vi "Main_Marvin.vi"() -> ()   [LabVIEW 2017]
uses:
  PCAN_Driver/ControlCAN.llb/DevType.ctl
  PCAN_Driver/ControlCAN.llb/CAN Channel.ctl
  PCAN_Driver/ControlCAN.llb/VCI_INIT_CONFIG.ctl
  PCAN_Driver/ControlCAN.llb/InitFlag.ctl
  PCAN_Driver/ControlCAN.llb/Fliter.ctl
  PCAN_Driver/ControlCAN.llb/Mode.ctl
  <vilib>/Utility/miscctls.llb/LVRowAndColumnTypeDef.ctl
  <vilib>/Utility/cursorutil.llb/Set Cursor (Icon Pict).vi
  PCAN_Driver/ControlCAN.lvlib
panel:
  in  "Stop Burn-in":bool
  out "Array 2":dbl[](array[numeric])
  out "VISA resource name out":refnum<visa-resource-name>
  out "UUT":u8
  out "CAN Status":bool
  in  "Channel 2":T1 caption="Channel" items=["Channel 1", "Channel 2"]
  out "Config_CANAT":T7 {"DevType" items=["USB-CAN"=3, "USB-CAN2"=4]; "CanIndex" items=["通道1", "通道2"]; "VCI_INIT_CONFIG"."Fliter" items=["接收所有类型"=3, "只接收标准帧"=4, "只接收扩展帧"=7]; "VCI_INIT_CONFIG"."Mode" items=["正常工作", "自测模式（环回）", "仅侦听模式"]; "VCI_INIT_CONFIG"."InitFlag" items=["使用Flash参数", "使用界面设置参数"]}
  out "Array":u64[][](array[numeric]) format="%016x"
  out "Motor Phase Current RMS":dbl
  out "Ambient Temperature":dbl
  out "Speed error":bool
  out "Commutation err":bool
  out "Under voltage/Over voltage":bool
  out "Derated drive temp":bool
  out "Motor Over temperature":bool
  out "Motor Sensor temp Fauilre":bool
  out "Drive Over temperature":bool
  out "Drive Sensor temp Failure":bool
  out "Ambient Over temp":bool
  out "Ambient Sensor temp":bool
  out "DC Voltage":dbl
  out "DC Current":dbl
  out "Power transistor Heat sink Temp.":dbl
  out "Motor Stator Temp.":dbl
  out "Motor Speed RPM":dbl
  out "ECS State":u16
  out "Waveform Chart":dbl[](graph)
  out "UUT":string="EBAY"
  in  "Logger Path":path
  in  "Report":bool
  in  "Start":bool
  out "Table Out":string[][](table)=[["Led -Test & On/Rst.Msg.", "", "", "", "", "", "", "", "", " ", "", "", "", "", " "], ["Led Test", "", "#1", "-", "-", "", "", "", "", " ", "", "", "", "", ""], ["Com.RS232 Rst.Msg", "", "#2", "-", "-", "", "", "", "", " ", "", "", "", "", ""], ["Com.RS232 Ans.Msg", "", "#3", "-", "-", "", "", "", "", "", "", "", "", "", ""], ["", "", "", "", "", "", "", "", "", "", "", "", "", "", ""], ["Servo Voltage & Current", "", "", "", "", "", "", "", "FAIL", "", "", "", "", "", ""], ["Servo Voltage", "", "28.0", "+/-1", "V", "", "NaN", "", "FAIL", "", "6.0", "0.0", "100", "Average", ""], ["Servo Current", "", "0.15", "Max", "A", "", "NaN", "", "FAIL", "", "1.0", "0.0", "100", "Average", ""], ["", "", "", "", "", "", "", "", "", "", "", "", "", "", ""], ["Voltages Accurance", "", "", "", "", "", "", "", "FAIL", "", "", "", "", "", ""], ["Servo VCC 5V    ", "", "5.0", "+/-0.1", "V", "", "NaN", "", "FAIL", "", "1.0", "0.0", "100", "Average", ""], ["Servo VEE -6.8V", "", "-6.8", "+/-0.15", "V", "", "NaN", "", "FAIL", "", "1.0", "0.0", "100", "Average", ""], ["Ref_1_4.096V ?", "", "4.096", "+/-0.1", "V", "", "NaN", "", "FAIL", "", "1.0", "0.0", "100", "Average", ""], ["", "", "", "", "", "", "", "", "", "", "", "", "", "", ""], ["Power-Supply Changing", "", "", "", "", "", "", "", "", "", "", "", "", "", ""], ["Min. Power-Supply Volt. 18v ", "", "Led Flashes", "-", "-", "", "", "", "", "", "", "", "", "", ""], ["Max. Power-Supply Volt. 32v ", "", "Led Flashes", "-", "-", "", "", "", "", "", "", "", "", "", ""], ["Under Volt.Prot.28->5->18v", "", "Led Flashes", "-", "-", "", "", "", "", "", "", "", "", "", ""], ["", "", "", "", "", "", "", "", "", "", "", "", "", "", ""], ["Pos.Cmd.Accur.@Mode1", "", "Mxxxx=", "", "", "", "", "", "", "", "", "", "", "", ""], ["Pos.Cmnd.=0.5V F.B.", "", "59h", "+/-5", "", "", "", "", "", "", "1.0", "0.0", "1", "Average", ""], ["Pos.Cmnd.=2.0V F.B.", "", "195h", "+/-5", "", "", "", "", "", "", "1.0", "0.0", "1", "Average", ""], ["Pos.Cmnd.=4.5V F.B.", "", "3A5h", "+/-5", "", "", "", "", "", "", "1.0", "0.0", "1", "Average", ""], ["", "", "", "", "", "", "", "", "", "", "", "", "", "", ""], ["Pos.Cmd.Accur.@Mode2", "", "Mxxxx=", "", "", "", "", "", "FAIL", "", "", "", "", "", ""], ["Pos.Cmnd.=0.5V F.B", "", "59h", "+/-5", "", "", "57h", "", "PASS", "", "1.0", "0.0", "1", "Average", ""], ["Pos.Cmnd.=2.0V F.B.", "", "195h", "+/-5", "", "", "1CEh", "", "FAIL", "", "1.0", "0.0", "1", "Average", ""], ["Pos.Cmnd.=4.5V F.B.", "", "3A5h", "+/-5", "", "", "2BAh", "", "FAIL", "", "1.0", "0.0", "1", "Average", ""], ["", "", "", "", "", "", "", "", "", "", "", "", "", "", ""], ["Pot.Accur.@Mode1 ", "", "Rxxxx=", "", "", "", "", "", "FAIL", "", "", "", "", "", ""], ["Pot.simulate=0.5v Pot.Code.:", "", "173h", "+/-5", "", "", "7Bh", "", "FAIL", "", "1.0", "0.0", "1", "Average", ""], ["Pot.simulate=2.0v Pot.Code.:", "", "1F3h", "+/-5", "", "", "1F1h", "", "PASS", "", "1.0", "0.0", "1", "Average", ""], ["Pot.simulate=3.5v Pot.Code.:", "", "372h", "+/-5", "", "", "368h", "", "FAIL", "", "1.0", "0.0", "1", "Average", ""], ["", "", "", "", "", "", "", "", "", "", "", "", "", "", ""], ["Pot.Accur.@Mode2 ", "", "Rxxxx=", "", "", "", "", "", "FAIL", "", "", "", "", "", ""], ["Pot.simulate=0.5v Pot.Code.:", "", "C4h", "+/-5", "", "", "7Bh", "", "FAIL", "", "1.0", "0.0", "1", "Average", ""], ["Pot.simulate=2.0v Pot.Code.:", "", "1E3h", "+/-5", "", "", "1F1h", "", "FAIL", "", "1.0", "0.0", "1", "Average", ""], ["Pot.simulate=3.5v Pot.Code.:", "", "541h", "+/-5", "", "", "368h", "", "FAIL", "", "1.0", "0.0", "1", "Average", ""], ["", "", "", "", "", "", "", "", "", "", "", "", "", "", ""], ["Status Accur.@Mode1", "", "", "", "", "", "", "", "", "", "", "", "", "", ""], ["Pot. / Pos.Cmnd. 1.5v", "", "-1.8084", "+/-0.1", "V", "", "", "", "", "", "1.0", "0.0", "100", "Average", ""], ["Pot. / Pos.Cmnd. 2.0v", "", "-0.1584", "+/-0.1", "V", "", "", "", "", "", "1.0", "0.0", "100", "Average", ""], ["Pot. / Pos.Cmnd. 3.5v", "", "4.7916", "+/-0.1", "V", "", "", "", "", "", "1.0", "0.0", "100", "Average", ""]]
  in  "ATR":string[][](table)=[["Test Communication", "-", "-", "-", "-", ""], ["Set S/N", "-", "-", "-", "-", ""], ["Set Board Number", "-", "-", "-", "-", ""], [" ", "", "", "", "", ""], ["Test Communication", "-", "-", "-", "-", ""], ["Get S/N", "-", "-", "-", "", ""], ["Get Board Number", "-", "-", "-", "", ""], ["Get FW", "-", "-", "-", "", ""], ["Enable Motor", "", "", "", "", ""], ["Small position command", "", "", "", "", ""], ["Measure delta", "", "", "", "", ""], ["Velocity command", "", "", "", "", ""]]
  in  "Settings":bool
  in  "Refresh Button":bool
  out "Status":bool
  in  "VISA resource name":refnum<visa-resource-name>="COM6"
  in  "Serial Com":bool
  in  "Help Button":bool
  out "Pannel User Message":string
  in  "Stop Button":bool
  # "Marvin"
  # "REDLER TECHNOLOGIES LTD"
  # "ver 1.0"
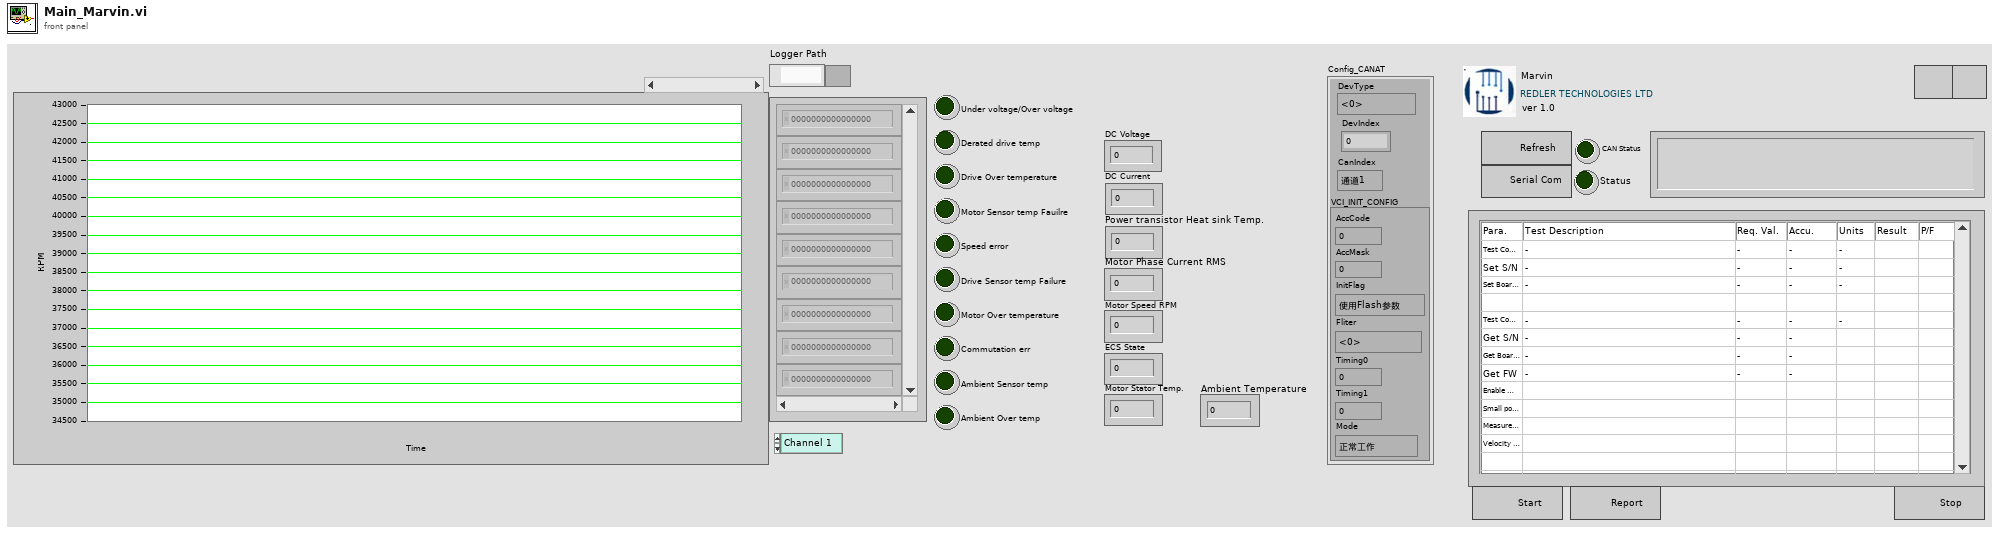
[diagram p1: front panel]
types:
  T1 = typedef "ControlCAN.lvlib/CAN Channel.ctl" = u32
  T2 = typedef "ControlCAN.lvlib/DevType.ctl" = u32
  T3 = typedef "ControlCAN.lvlib/VCI_INIT_CONFIG.ctl" = cluster{"AccCode":u32, "AccMask":u32, "InitFlag":T4, "Fliter":T5, "Timing0":u8, "Timing1":u8, "Mode":T6}
  T4 = typedef "ControlCAN.lvlib/InitFlag.ctl" = u32
  T5 = typedef "ControlCAN.lvlib/Fliter.ctl" = u8
  T6 = typedef "ControlCAN.lvlib/Mode.ctl" = u8
  T7 = cluster{"DevType":T2, "DevIndex":u32, "CanIndex":T1, "VCI_INIT_CONFIG":T3}
  T8 = cluster{"VISA":refnum<visa-resource-name>, "Array Test":enum16{"Auxiliary", "Temp Sens Cal", "Com Test", "Enable Test", "Speed Command", "Stop Time", "Temp Control", "Burn in", "Visual Inspec", "Empty"}[]}
  T9 = cluster{"ID":u32, "MSGTYPE":u8, "LEN":u8, "aDATA":u8[]}[]
  T10 = enum16{"Erase ATR Table", "Stop", "MainProgram", "Initialize"}
  T11 = enum16{"Auxiliary", "Temp Sens Cal", "Com Test", "Enable Test", "Speed Command", "Stop Time", "Temp Control", "Burn in", "Visual Inspec", "Empty"}[]
  T12 = typedef "LVRowAndColumnTypeDef.ctl" = cluster{"Row":i32, "Column":i32}
  T13 = cluster{"ID":u32, "MSGTYPE":u8, "LEN":u8, "aDATA":u8[]}
  T14 = enum16{"Auxiliary", "Temp Sens Cal", "Com Test", "Enable Test", "Speed Command", "Stop Time", "Temp Control", "Burn in", "Visual Inspec", "Empty"}
  T15 = enum16{"open", "replace", "create", "open or create", "replace or create", "replace or create with confirmation"}
  T16 = enum32{"Invalid", "Standard", "Closed", "Hidden", "Minimized", "Maximized"}
  T17 = typedef "ControlCAN.lvlib/VCI_CAN_OBJ.ctl" = cluster{"ID":u32, "TimeStamp":u32, "TimeFlag":u8, "SendType":u8, "RemoteFlag":u8, "ExternFlag":u8, "DataLen":u8, "Data":u8[], "Reserved":u8[]}
  T18 = cluster{"Type":enum16{"接收", "发送"}, "Channel":T1, "Time":timestamp, "VCI_CAN_OBJ":T17}[]
  T19 = cluster{"Type":enum16{"接收", "发送"}, "Channel":T1, "Time":timestamp, "VCI_CAN_OBJ":T17}
  T20 = typedef "LVPoint32TypeDef.ctl" = cluster{"Horizontal":i32, "Vertical":i32}
  T21 = enum16{"Visual Inspection", "Temp Sens Cal", "Com Test", "Enable Test", "Speed Command", "Stop Time", "Temp Control", "Burn in", "Visual Inspec", "Empty"}[]
  T22 = enum16{"Auxiliary", "Temp Sens Cal", "Com Test", "Enable Test", "Speed Command", "Stop Time", "Burn in", "Visual Inspec", "Empty"}[]
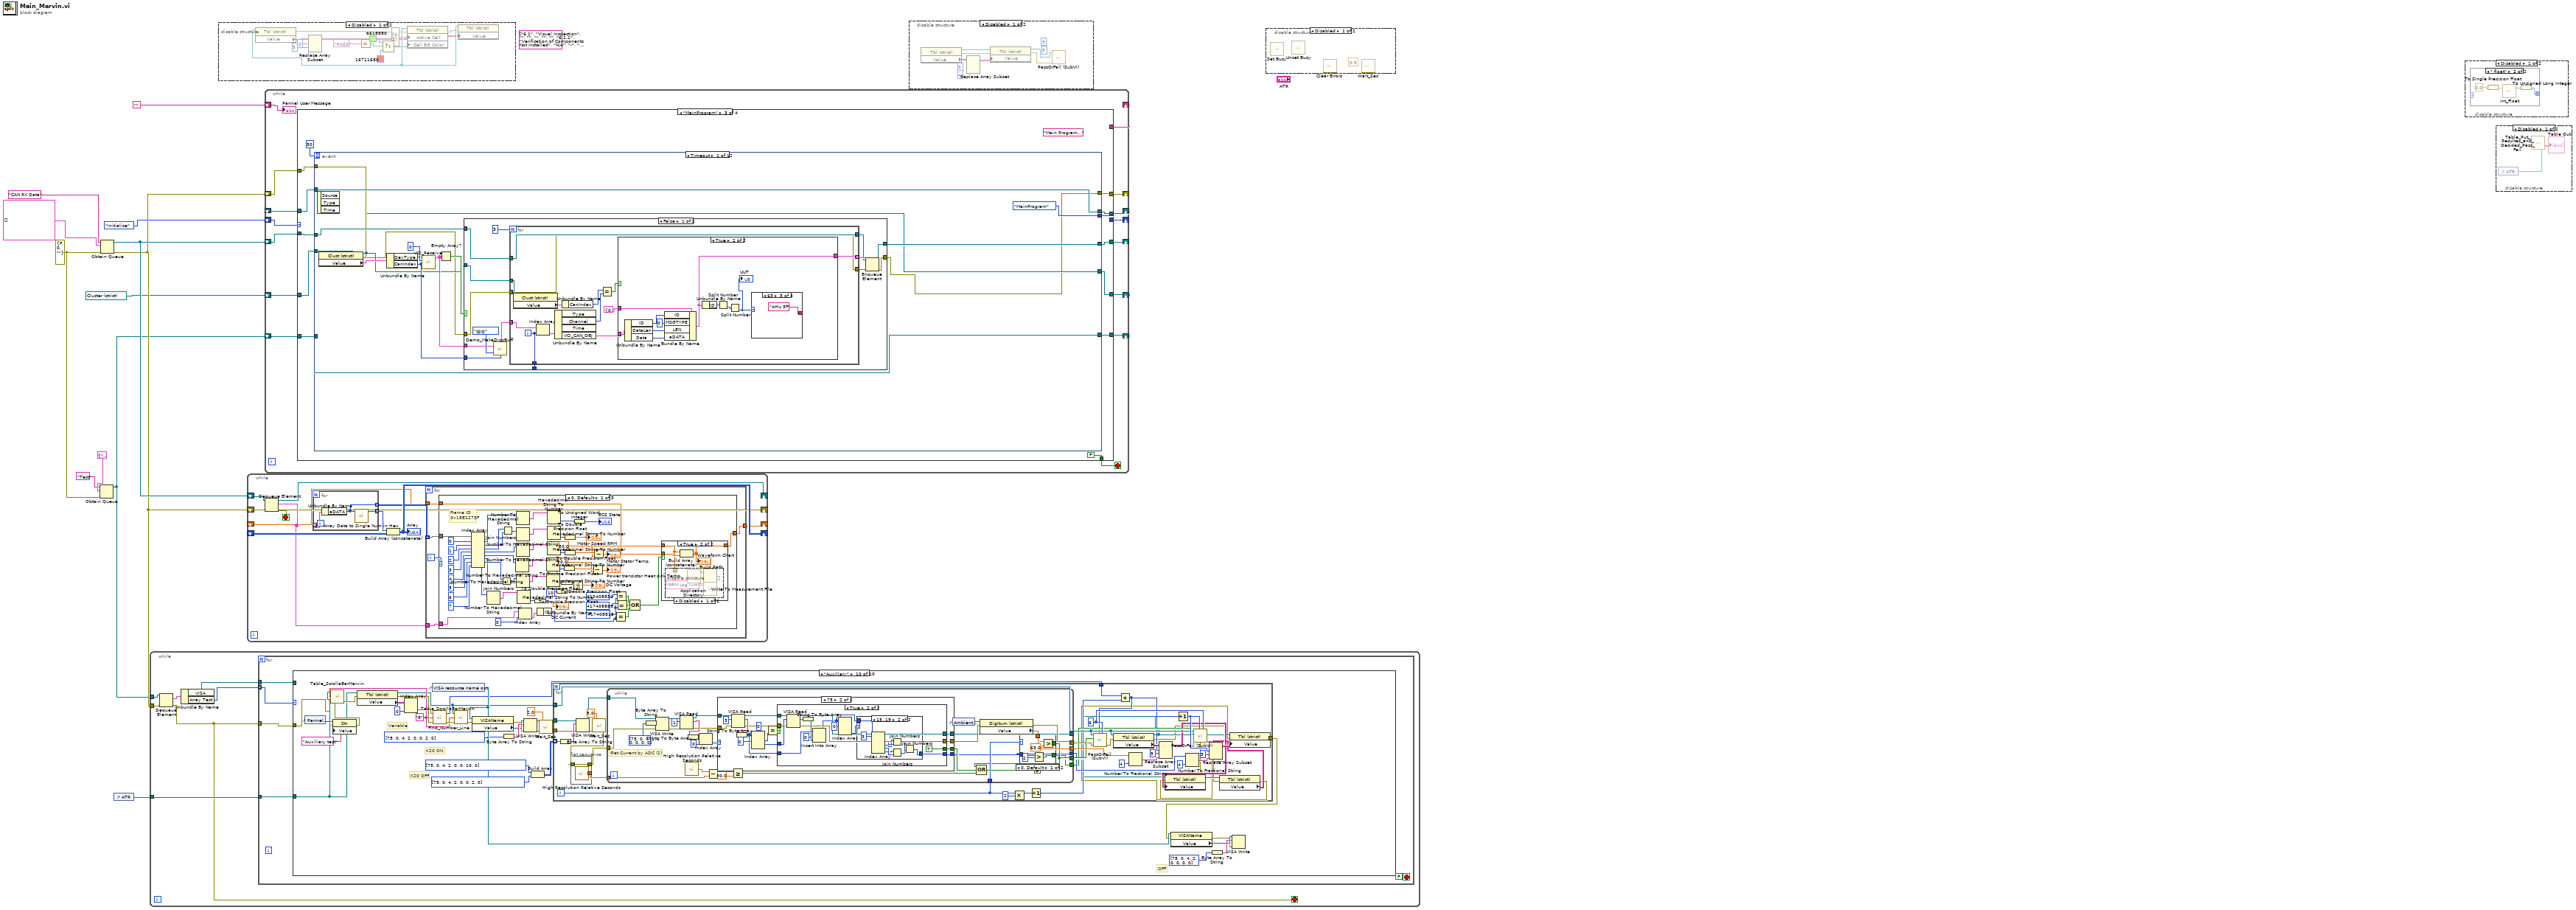
[diagram p0: block diagram]
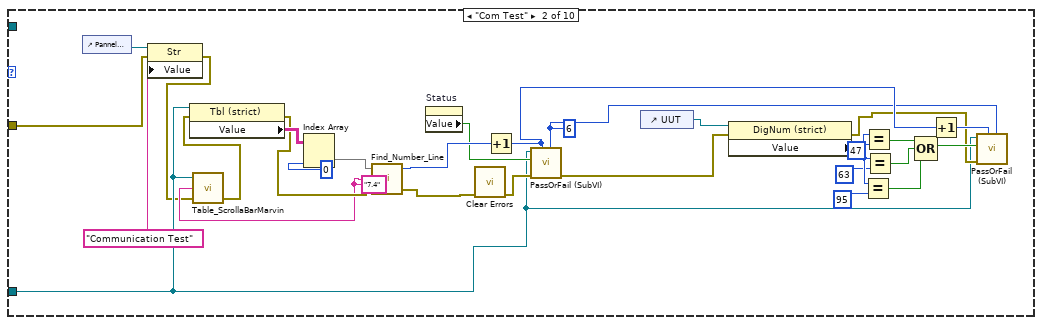
[diagram p3: hidden frame]
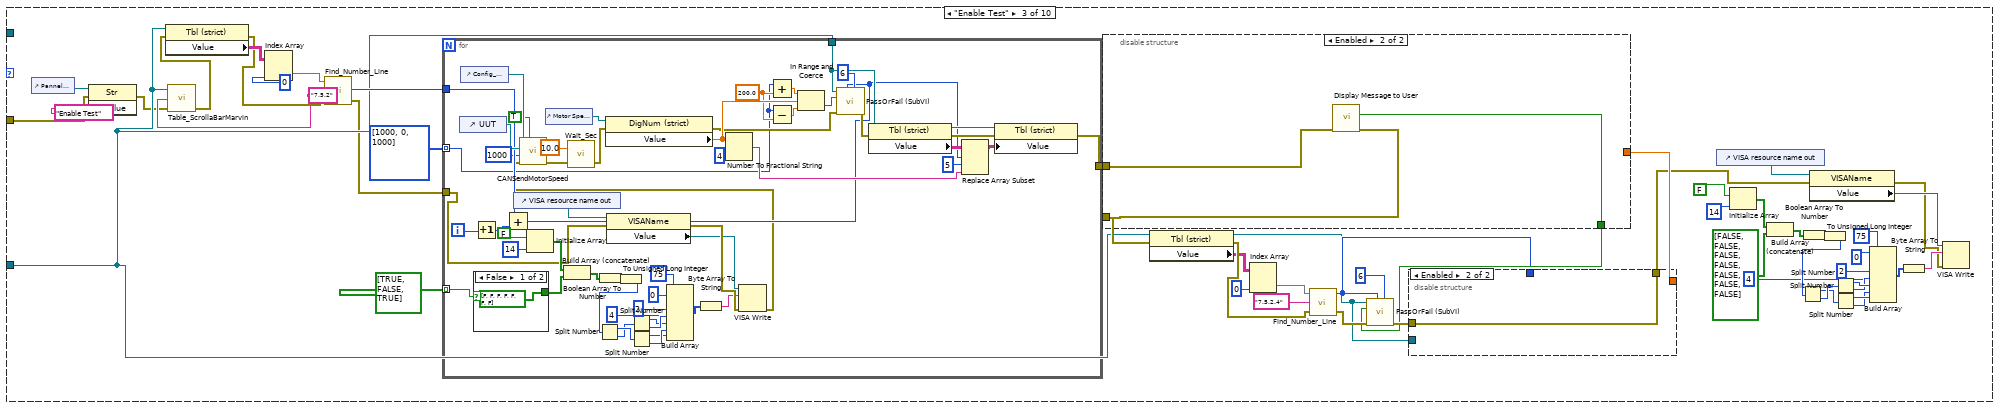
[diagram p4: hidden frame]
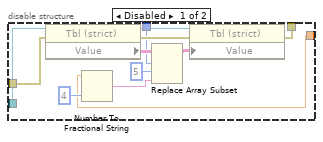
[diagram p5: hidden frame]
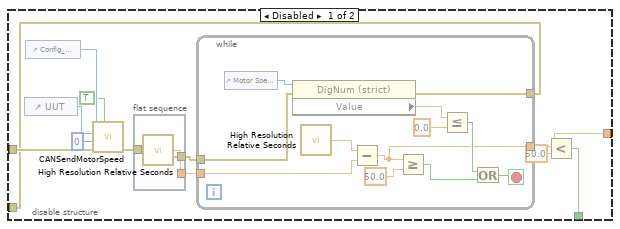
[diagram p6: hidden frame]
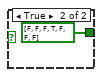
[diagram p7: hidden frame]
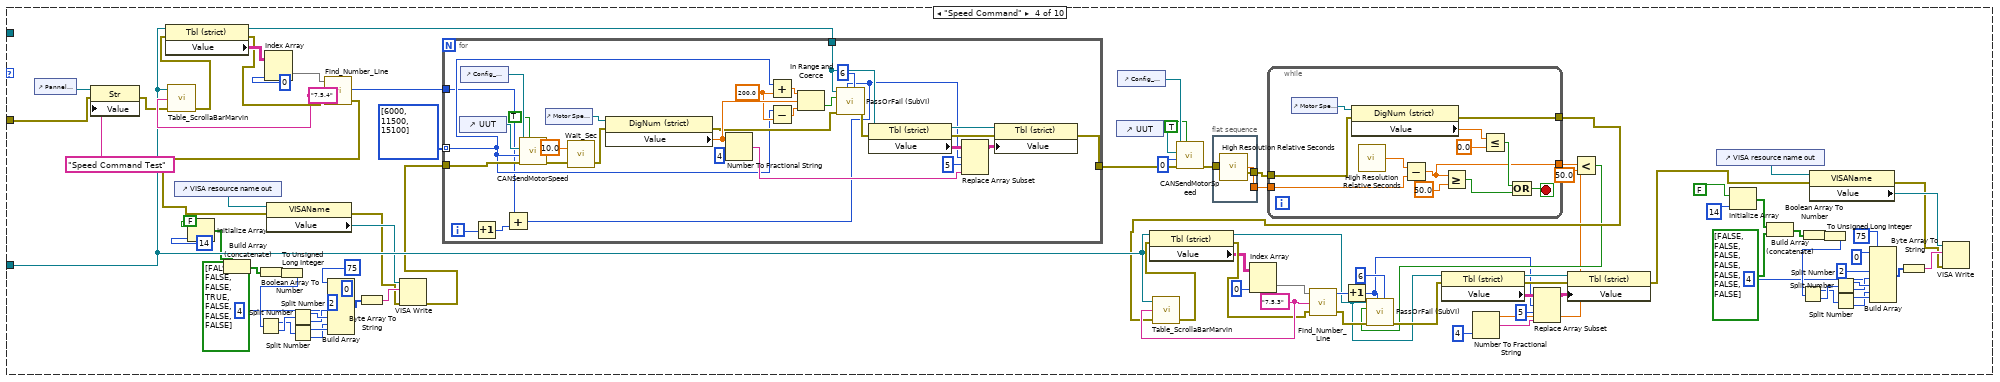
[diagram p8: hidden frame]
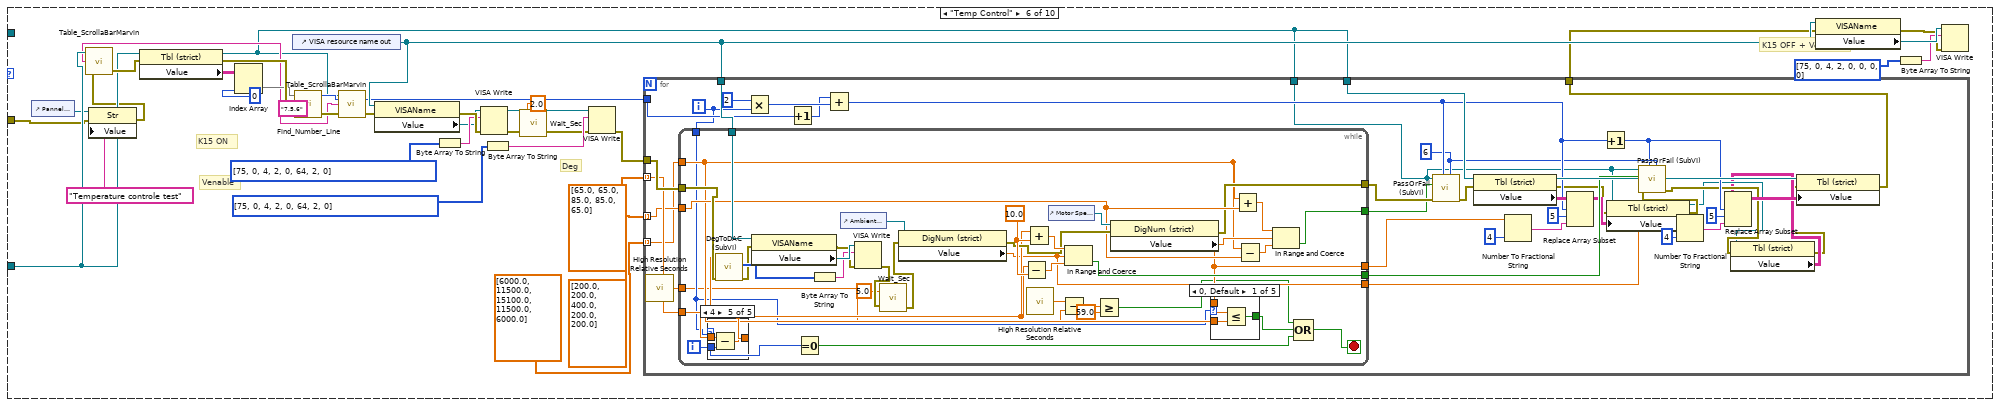
[diagram p10: hidden frame]
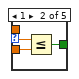
[diagram p11: hidden frame]
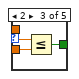
[diagram p12: hidden frame]
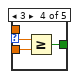
[diagram p13: hidden frame]
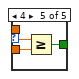
[diagram p14: hidden frame]
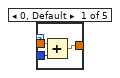
[diagram p15: hidden frame]
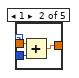
[diagram p16: hidden frame]
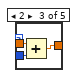
[diagram p17: hidden frame]
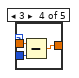
[diagram p18: hidden frame]
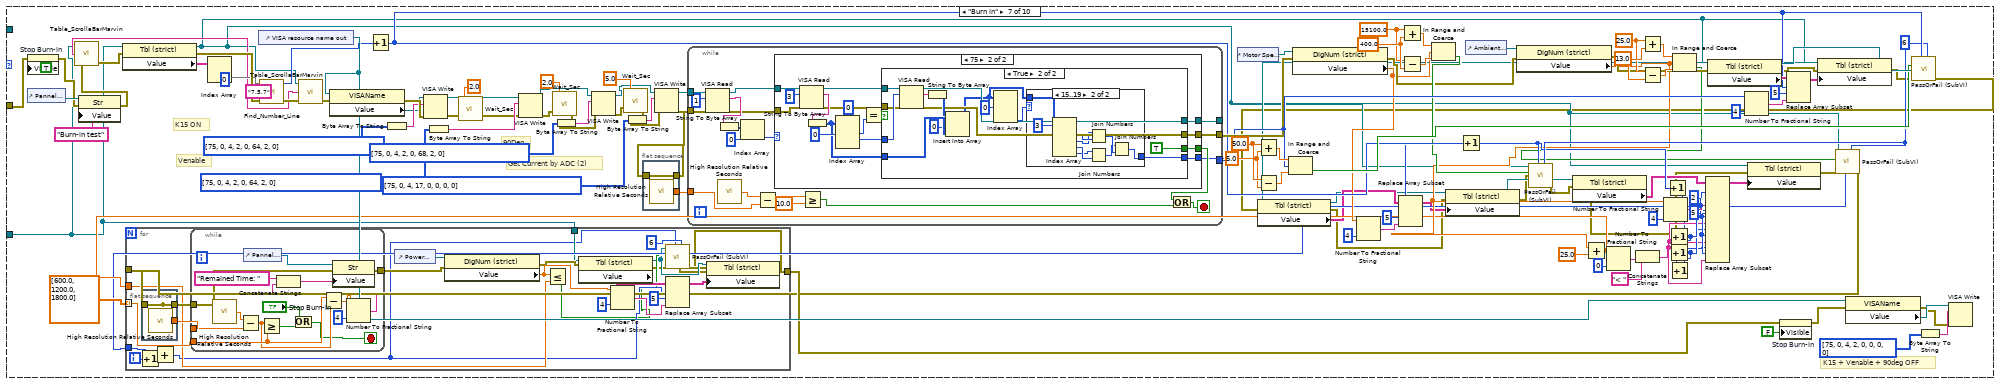
[diagram p19: hidden frame]
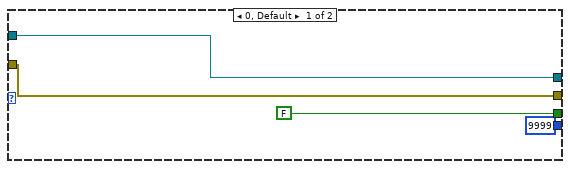
[diagram p20: hidden frame]
diagram:
  w6 = errorcluster {"status"=FALSE, "code"=0, "source"=""} ("error in (no error)")
  (unwired) string[][] [["6.1", "Visual Inspection", "", "", "", "", ""], ["6.1.1", "Verification of Components Not Installed", "N/A", "-", "", "", ""], ["", "", "", "", "", "", ""], ["6.1.2", "Manufacturing Defects", "N/A", "-", "", "", ""], ["", "", "", "", "", "", ""], ["6.2", "Power Supply Testing", "", "", "", "", ""], ["6.2.1", "Input Current Drawn", "", "", "", "", ""], ["6.2.1.1", "DC Input Current", "< 150", "-", "mA", "", ""], ["", "", "", "", "", "", ""], ["6.2.2", "Power Supply Voltages", "", "", "", "", ""], ["6.2.2.1", "12V", "12.0", "+/-0.500", "V", "", ""], ["6.2.2.2", "5V", "5.0", "+/-0.200", "V", "", ""], ["6.2.2.3", "3.3V", "3.3", "+/-0.100", "V", "", ""], ["6.2.2.4", "1.8V", "1.8", "+/-0.100", "V", "", ""], ["", "", "", "", "", "", ""], ["7", "Functional Test Procedure", "", "", "", "", ""], ["7.1", "Weight Check", "4180", "+/-10.00", "gr", "", ""], ["", "", "", "", "", "", ""], ["7.2", "Insulation Resistance Test", "", "", "", "", ""], ["7.2.1", "J3.B to Chassis", "> 1M", "-", "ohms", "", ""], ["7.2.2", "J1.16 to Chassis", "> 100K", "-", "ohms", "", ""], ["", "", "", "", "", "", ""], ["7.2", "Bonding Resistance", "", "", "", "", ""], ["7.2.3", "J1 Body to Chassis", "< 2m", "-", "ohms", "", ""], ["7.2.4", "J2  Body to Chassis", "< 2m", "-", "ohms", "", ""], ["7.2.5", "J3  Body to Chassis", "< 2m", "-", "ohms", "", ""], ["", "", "", "", "", "", ""], ["7.2.1", "CANbus Resistance Test", "", "", "", "", ""], ["7.2.1.1", "J1.17 to J1.18", "> 10K", "-", "ohms", "", ""], ["", "", "", "", "", "", ""], ["7.3", "Sealing Test", "N/A", "-", "", "", ""], ["", "", "", "", "", "", ""], ["7.4", "Communication Test", "", "", "", "", ""], ["7.4.1", "Serial RS-232", "N/A", "-", "", "", ""], ["7.4.2", "CAN Bus", "N/A", "-", "", "", ""], ["", "", "", "", "", "", ""], ["7.5", "Performances Tests", "", "", "", "", ""], ["7.5.1", "Reverse Polarity Test", "", "", "", "", ""], ["7.5.1.1", "DC Input Current", "< 1", "-", "mA", "", ""], ["", "", "", "", "", "", ""], ["7.5.2", "Enable Test", "", "", "", "", ""], ["7.5.2.1", "Fan Speed at Opened Enable ", "0", "-", "rpm", "", ""], ["7.5.2.2", "Fan Speed at Closed Enable ", "6000", "+/-200.0", "rpm", "", ""], ["7.5.2.3", "Motor Rotation Direction", "Counter-clockwise (Inlet)", "-", "", "", ""], ["", "", "", "", "", "", ""], ["7.5.3", "Stop Time Test ", "", "", "", "", ""], ["7.5.3.1", "Motor Stop time", "< 50", "-", "sec", "", ""], ["", "", "", "", "", "", ""], ["7.5.4", "Speed Command Test", "", "", "", "", ""], ["7.5.4.1", "Fan Speed", "6000", "+/-200.0", "rpm", "", ""], ["7.5.4.2", "Fan Speed", "11500", "+/-200.0", "rpm", "", ""], ["7.5.4.3", "Fan Speed", "15100", "+/-200.0", "rpm", "", ""], ["", "", "", "", "", "", ""], ["7.5.5", "Temperature Sensor Calibration Test", "", "", "", "", ""], ["7.5.5.1", "Sensor Reading Analog Offset", "0", "+/-0.100", ".", "", ""], ["", "", "", "", "", "", ""], ["7.5.6", "Temperature Control Algorithm Test", "", "", "", "", ""], ["7.5.6.1", "Tair <   68 ± 2 oC", "6000", "+/-200.0", "rpm", "", ""], ["7.5.6.2", "Tair >= 68 ± 2 oC", "11500", "+/-200.0", "rpm", "", ""], ["7.5.6.3", "Tair >= 88 ± 2 oC", "15100", "+/-400.0", "rpm", "", ""], ["7.5.6.4", "Tair <= 80 ± 2 oC", "11500", "+/-200.0", "rpm", "", ""], ["7.5.6.5", "Tair <= 60 ± 2 oC", "6000", "+/-200.0", "rpm", "", ""], ["", "", "", "", "", "", ""], ["7.5.7", "Burn-in Test", "", "", "", "", ""], ["7.5.7.1", "DC Input Current", "50", "+/-5.000", "A", "", ""], ["7.5.7.2", "Ambient Temperature", "25", "+/-13.00", "Deg.", "", ""], ["7.5.7.3", "After 10 min of operation", "", "", "Deg.", "", ""], ["7.5.7.4", "After 20 min of operation", "", "", "Deg.", "", ""], ["7.5.7.5", "After 30 min of operation", "", "", "Deg.", "", ""], ["7.5.7.6", "Auxiliary Cooling Fan 60 Deg", "On", "-", ".", "", ""], ["7.5.7.7", "Auxiliary Cooling Fan 55 Deg", "Off", "-", ".", "", ""]] ("data")
  n1 = Obtain Queue(name (unnamed)="Test", element data type=T8 {"VISA"="COM1", "Array Test"=[]}, error in (no error)=w6) -> (queue out=w3:refnum<queue>)  [unwired: 2 in, 2 out]
  n2 = Obtain Queue(name (unnamed)="CAN RX Data", element data type=T9 [], error in (no error)=w6) -> (queue out=w8:refnum<queue>, error out=w4:errorcluster)  [unwired: 2 in, 1 out]
  n3 = control-ref of="ATR"() -> (w5:refnum<vi>)
  n4 = while {
    tunnel: w5 -> [w19]
    tunnel: w4 -> [w17]
    tunnel: w3 -> [w18]
    stop <- w13 stop-if-true
    n5 = Dequeue Element(queue=w18, error in (no error)=w17) -> (element=w16:T8, error out=w13:errorcluster)  [unwired: 1 in, 2 out]
    n6 = Unbundle By Name(w16) -> ("VISA"=w15:refnum<visa-resource-name>, "Array Test"=w14:T11)
    n7 = for {
      tunnel: w14 -> [w20] mode=indexing
      tunnel: w15 -> [w24]
      tunnel: w19 -> [w23]
      tunnel: w13 -> [w22]
      stop <- FALSE stop-if-true
      n8 = case shown="\"Auxiliary\"" w20 {
        tunnel: w24 -> [_ _ _ _ _ _ _ _ w717 _]
        tunnel: w23 -> [_ w31 w60 w272 _ w366 w502 w709 w726 w839]
        tunnel: w22 -> [_ w27 w56 w207 _ w344 w507 w710 w713 w838]
        frame "Empty", Default {
        }
        frame "Com Test" {
          w32 = 6 ("disabled index (col)")
          w30 = "7.4" ("Test Paragraph")
          n9 = control-ref of="Pannel User Message"() -> (w28:refnum<vi>)
          n10 = property class="Str"(reference=w28, error in=w27, "Value"="Communication Test") -> (error out=w26:errorcluster)  [unwired: 1 out]
          n11 = call "Table_ScrollaBarMarvin.vi"("error in"=w26, "Line to focus"=w30, "reference in"=w31) -> ("error out"=w29:errorcluster)  [unwired: 2 out]
          n12 = property class="Tbl (strict)"(reference=w31, error in=w29) -> (error out=w51:errorcluster, "Value"=w52:string[][])  [unwired: 1 out]
          n13 = Index Array(array=w52, index (col)=0 ("disabled index (col)")) -> (element=w53:string[])  [unwired: 1 in]
          n14 = call "Find_Number_Line.vi"("error in"=w51, "Test Paragraph"=w30, "Row Headers[]"=w53) -> ("error out"=w49:errorcluster, "Line number"=w48:i32)  [unwired: 1 out]
          n15 = property on="Status" class="Bool (strict)"() -> ("Value"=w46:bool)  [unwired: 2 in, 2 out]
          n16 = call <vilib>:"Clear Errors.vi"("error in (no error)"=w49) -> ("error out"=w47:errorcluster)  [unwired: 5 in, 1 out]
          n17 = Increment(x=w48) -> (x+1=w36:i32)
          n18 = call "PassOrFail (SubVI).vi"("disabled index (col)"=w32, "index (row)"=w36, "error in (no error)"=w47, "Boolean"=w46, "Table in"=w31) -> ("error out"=w44:errorcluster)  [unwired: 6 in]
          n19 = control-ref of="UUT"() -> (w45:refnum<vi>)
          n20 = property class="DigNum (strict)"(reference=w45, error in=w44) -> (error out=w33:errorcluster, "Value"=w43:u8)  [unwired: 1 out]
          n21 = Equal?(x=w43, y=u8 95) -> (x = y?=w37:bool)
          n22 = Equal?(x=w43, y=u8 47) -> (x = y?=w39:bool)
          n23 = Equal?(x=w43, y=u8 63) -> (x = y?=w38:bool)
          n24 = Compound Arithmetic op=OR(w39, w38, w37) -> (w34:bool)
          n25 = Increment(x=w36) -> (x+1=w35:i32)
          n26 = call "PassOrFail (SubVI).vi"("disabled index (col)"=w32, "index (row)"=w35, "error in (no error)"=w33, "Boolean"=w34, "Table in"=w31) -> ()  [unwired: 6 in, 1 out]
        }
        frame "Enable Test" {
          w101 = "7.5.2" ("Test Paragraph")
          n27 = control-ref of="Pannel User Message"() -> (w57:refnum<vi>)
          n28 = property class="Str"(reference=w57, error in=w56, "Value"="Enable Test") -> (error out=w55:errorcluster)  [unwired: 1 out]
          n29 = call "Table_ScrollaBarMarvin.vi"("error in"=w55, "Line to focus"=w101, "reference in"=w60) -> ("error out"=w100:errorcluster)  [unwired: 2 out]
          n30 = property class="Tbl (strict)"(reference=w60, error in=w100) -> (error out=w103:errorcluster, "Value"=w104:string[][])  [unwired: 1 out]
          n31 = Index Array(array=w104, index (col)=0 ("disabled index (col)")) -> (element=w105:string[])  [unwired: 1 in]
          n32 = call "Find_Number_Line.vi"("error in"=w103, "Test Paragraph"=w101, "Row Headers[]"=w105) -> ("error out"=w59:errorcluster, "Line number"=w99:i32)  [unwired: 1 out]
          n33 = for {
            tunnel: w60 -> [w191]
            tunnel: w99 -> [w181]
            tunnel: u16[] [1000, 0, 1000] -> [w150] mode=indexing
            tunnel: [w177] -> w97
            tunnel: w59 -> [w151]
            tunnel: bool[] [TRUE, FALSE, TRUE] -> [w148] mode=indexing
            i -> [w183]
            w184 = 200.0 ("y")
            n34 = control-ref of="UUT"() -> (w202:refnum<vi>)
            n35 = control-ref of="Config_CANAT"() -> (w201:refnum<vi>)
            n36 = Increment(x=w183) -> (x+1=w182:i32)
            n37 = case shown="False" w148 {
              tunnel: [bool[] [FALSE, FALSE, FALSE, FALSE, FALSE, FALSE, FALSE] ("array") bool[] [FALSE, FALSE, FALSE, TRUE, FALSE, FALSE, FALSE] ("array")] -> w159
              frame False {
              }
              frame True {
              }
            }
            n38 = Add(x=w181, y=w182) -> (x+y=w176:i32)
            n39 = control-ref of="VISA resource name out"() -> (w173:refnum<vi>)
            n40 = Initialize Array(FALSE, 14 ("dimension size")) -> (w161:bool[])
            n41 = control-ref of="Motor Speed RPM"() -> (w200:refnum<vi>)
            n42 = Build Array (concatenate)(w161, w159) -> (w160:bool[])
            n43 = Boolean Array To Number(Boolean array=w160) -> (number=w162:u32)
            n44 = property class="VISAName"(reference=w173, error in=w151) -> (error out=w174:errorcluster, "Value"=w164:refnum<visa-resource-name>)  [unwired: 1 out]
            n45 = To Unsigned Long Integer(number=w162) -> (unsigned 32bit integer=w171:u32)
            n46 = Split Number(x=w171) -> (hi(x)=w166:u16, lo(x)=w165:u16)
            n47 = Split Number(x=w165) -> (hi(x)=w167:u8, lo(x)=w168:u8)
            n48 = Split Number(x=w166) -> (hi(x)=w169:u8, lo(x)=w170:u8)
            n49 = Build Array(u8 75, u8 0 ("element"), u8 4 ("Length"), u8 2, w168, w167, w170, w169) -> (w163:u8[])
            n50 = Byte Array To String(unsigned byte array=w163) -> (string=w172:string)
            n51 = VISA Write(VISA resource name=w164, write buffer=w172, error in (no error)=w174) -> (error out=w152:errorcluster)  [unwired: 2 out]
            n52 = call "CANSendMotorSpeed.vi"("Remote"=TRUE, "error in (no error)"=w152, "Motor Speed RPM"=u16 1000, "UUT"=w202, "Cluster in"=w201) -> ("error out"=w198:errorcluster)  [unwired: 6 in]
            n53 = call "Wait_Sec.vi"("Delay Time (sec)"=10.0, "error out"=w198) -> ("error in"=w179:errorcluster)  [unwired: 2 in]
            n54 = property class="DigNum (strict)"(reference=w200, error in=w179) -> (error out=w193:errorcluster, "Value"=w194:dbl)  [unwired: 1 out]
            n55 = Number To Fractional String(number=w194, precision (6)=i16 4) -> (F-format string=w190:string)  [unwired: 2 in]
            n56 = Add(x=w150, y=w184) -> (x+y=w186:dbl)
            n57 = Subtract(x=w150, y=w184) -> (x-y=w185:dbl)
            n58 = In Range and Coerce(upper limit=w186, x=w194, lower limit=w185) -> (In Range?=w192:bool)  [unwired: 1 out]
            n59 = call "PassOrFail (SubVI).vi"("disabled index (col)"=6, "index (row)"=w176, "error in (no error)"=w193, "Boolean"=w192, "Table in"=w191) -> ("error out"=w196:errorcluster)  [unwired: 6 in]
            n60 = property class="Tbl (strict)"(reference=w191, error in=w196) -> (reference out=w187:refnum<vi>, error out=w197:errorcluster, "Value"=w188:string[][])
            n61 = Replace Array Subset(array=w188, new element=w190, index (row)=w176, index (col)=5 ("disabled index (col)")) -> (w189:string[][])
            n62 = property class="Tbl (strict)"(reference=w187, error in=w197, "Value"=w189) -> (error out=w177:errorcluster)  [unwired: 1 out]
          }
          n63 = disable-structure shown="Enabled" {
            disable-tunnel: w97 -> [w128 w146]
            disable-tunnel: [w123 w145] -> w90
            disable-tunnel: [w121 w147] -> w87
            disable-tunnel: [w120 _] -> w85
            frame Disabled {
              n64 = control-ref of="UUT"() -> (w129:refnum<vi>)
              n65 = control-ref of="Config_CANAT"() -> (w130:refnum<vi>)
              n66 = call "CANSendMotorSpeed.vi"("Remote"=TRUE, "error in (no error)"=w128, "Motor Speed RPM"=u16 0, "UUT"=w129, "Cluster in"=w130) -> ("error out"=w125:errorcluster)  [unwired: 6 in]
              n67 = flat-sequence {
                tunnel: [w132] -> w126
                tunnel: w125 -> [w131]
                tunnel: [w131] -> w124
                frame #0 {
                  n68 = call <vilib>:"High Resolution Relative Seconds.vi"() -> ("relative seconds"=w132:dbl)
                }
              }
              n69 = while {
                tunnel: w126 -> [w140]
                tunnel: w124 -> [w133]
                tunnel: [w135] -> w120
                tunnel: [w134] -> w123
                stop <- w138 stop-if-true
                n70 = control-ref of="Motor Speed RPM"() -> (w144:refnum<vi>)
                n71 = property class="DigNum (strict)"(reference=w144, error in=w133) -> (error out=w134:errorcluster, "Value"=w143:dbl)  [unwired: 1 out]
                n72 = call <vilib>:"High Resolution Relative Seconds.vi"() -> ("relative seconds"=w141:dbl)
                n73 = Subtract(x=w141, y=w140) -> (x-y=w135:dbl)
                n74 = Greater Or Equal?(x=w135, y=50.0) -> (x >= y?=w136:bool)
                n75 = Less Or Equal?(x=w143, y=0.0) -> (x <= y?=w137:bool)
                n76 = Or(x=w137, y=w136) -> (x .or. y?=w138:bool)
              }
              n77 = Less?(x=w120, y=50.0) -> (x < y?=w121:bool)
            }
            frame Enabled {
              n78 = call "Display Message to User"("error in (no error)"=w146) -> ("error out"=w145:errorcluster, "YES"=w147:bool)  [unwired: 9 in]
            }
          }
          n79 = property class="Tbl (strict)"(reference=w60, error in=w90) -> (reference out=w84:refnum<vi>, error out=w94:errorcluster, "Value"=w93:string[][])
          n80 = Index Array(array=w93, index (col)=0 ("disabled index (col)")) -> (element=w92:string[])  [unwired: 1 in]
          n81 = call "Find_Number_Line.vi"("error in"=w94, "Test Paragraph"="7.5.2.4", "Row Headers[]"=w92) -> ("error out"=w91:errorcluster, "Line number"=w86:i32)  [unwired: 1 out]
          n82 = call "PassOrFail (SubVI).vi"("disabled index (col)"=6, "index (row)"=w86, "error in (no error)"=w91, "Boolean"=w87, "Table in"=w84) -> ("error out"=w88:errorcluster)  [unwired: 6 in]
          n83 = disable-structure shown="Enabled" {
            disable-tunnel: w88 -> [w112 w118]
            disable-tunnel: w86 -> [w109 _]
            disable-tunnel: w85 -> [w108 _]
            disable-tunnel: w84 -> [w107 _]
            disable-tunnel: [w106 w118] -> w61
            frame Disabled {
              n84 = property class="Tbl (strict)"(reference=w107, error in=w112) -> (reference out=w117:refnum<vi>, error out=w113:errorcluster, "Value"=w116:string[][])
              n85 = Number To Fractional String(number=w108, precision (6)=i16 4) -> (F-format string=w110:string)  [unwired: 2 in]
              n86 = Replace Array Subset(array=w116, new element=w110, index (row)=w109, index (col)=5 ("disabled index (col)")) -> (w115:string[][])
              n87 = property class="Tbl (strict)"(reference=w117, error in=w113, "Value"=w115) -> (error out=w106:errorcluster)  [unwired: 1 out]
            }
            frame Enabled {
            }
          }
          n88 = control-ref of="VISA resource name out"() -> (w70:refnum<vi>)
          n89 = Initialize Array(FALSE, 14 ("dimension size")) -> (w82:bool[])
          n90 = Build Array (concatenate)(w82, bool[] [FALSE, FALSE, FALSE, FALSE, FALSE, FALSE, FALSE] ("array")) -> (w83:bool[])
          n91 = Boolean Array To Number(Boolean array=w83) -> (number=w81:u32)
          n92 = property class="VISAName"(reference=w70, error in=w61) -> (error out=w69:errorcluster, "Value"=w79:refnum<visa-resource-name>)  [unwired: 1 out]
          n93 = To Unsigned Long Integer(number=w81) -> (unsigned 32bit integer=w72:u32)
          n94 = Split Number(x=w72) -> (hi(x)=w77:u16, lo(x)=w78:u16)
          n95 = Split Number(x=w78) -> (hi(x)=w76:u8, lo(x)=w75:u8)
          n96 = Split Number(x=w77) -> (hi(x)=w74:u8, lo(x)=w73:u8)
          n97 = Build Array(u8 75, u8 0 ("element"), u8 4 ("Length"), u8 2, w75, w76, w73, w74) -> (w80:u8[])
          n98 = Byte Array To String(unsigned byte array=w80) -> (string=w71:string)
          n99 = VISA Write(VISA resource name=w79, write buffer=w71, error in (no error)=w69) -> ()  [unwired: 3 out]
        }
        frame "Speed Command" {
          w279 = "7.5.3" ("Test Paragraph")
          w291 = "7.5.4" ("Test Paragraph")
          n100 = control-ref of="Pannel User Message"() -> (w208:refnum<vi>)
          n101 = property class="Str"(reference=w208, error in=w207, "Value"="Speed Command Test") -> (error out=w206:errorcluster)  [unwired: 1 out]
          n102 = call "Table_ScrollaBarMarvin.vi"("error in"=w206, "Line to focus"=w291, "reference in"=w272) -> ("error out"=w290:errorcluster)  [unwired: 2 out]
          n103 = property class="Tbl (strict)"(reference=w272, error in=w290) -> (error out=w293:errorcluster, "Value"=w294:string[][])  [unwired: 1 out]
          n104 = control-ref of="VISA resource name out"() -> (w243:refnum<vi>)
          n105 = Initialize Array(FALSE, 14 ("dimension size")) -> (w255:bool[])
          n106 = Build Array (concatenate)(w255, bool[] [FALSE, FALSE, FALSE, TRUE, FALSE, FALSE, FALSE] ("array")) -> (w256:bool[])
          n107 = Boolean Array To Number(Boolean array=w256) -> (number=w254:u32)
          n108 = Index Array(array=w294, index (col)=0 ("disabled index (col)")) -> (element=w295:string[])  [unwired: 1 in]
          n109 = To Unsigned Long Integer(number=w254) -> (unsigned 32bit integer=w245:u32)
          n110 = Split Number(x=w245) -> (hi(x)=w250:u16, lo(x)=w251:u16)
          n111 = Split Number(x=w251) -> (hi(x)=w249:u8, lo(x)=w248:u8)
          n112 = Split Number(x=w250) -> (hi(x)=w247:u8, lo(x)=w246:u8)
          n113 = call "Find_Number_Line.vi"("error in"=w293, "Test Paragraph"=w291, "Row Headers[]"=w295) -> ("error out"=w234:errorcluster, "Line number"=w289:i32)  [unwired: 1 out]
          n114 = property class="VISAName"(reference=w243, error in=w234) -> (error out=w242:errorcluster, "Value"=w252:refnum<visa-resource-name>)  [unwired: 1 out]
          n115 = Build Array(u8 75, u8 0 ("element"), u8 4 ("Length"), u8 2, w248, w249, w246, w247) -> (w253:u8[])
          n116 = Byte Array To String(unsigned byte array=w253) -> (string=w244:string)
          n117 = VISA Write(VISA resource name=w252, write buffer=w244, error in (no error)=w242) -> (error out=w233:errorcluster)  [unwired: 2 out]
          n118 = for {
            tunnel: w233 -> [w331]
            tunnel: w272 -> [w327]
            tunnel: w289 -> [w316]
            tunnel: u16[] [6000, 11500, 15100] -> [w319] mode=indexing
            tunnel: [w312] -> w285
            i -> [w318]
            w320 = 200.0 ("y")
            n119 = control-ref of="UUT"() -> (w339:refnum<vi>)
            n120 = control-ref of="Config_CANAT"() -> (w338:refnum<vi>)
            n121 = Increment(x=w318) -> (x+1=w317:i32)
            n122 = Add(x=w316, y=w317) -> (x+y=w311:i32)
            n123 = call "CANSendMotorSpeed.vi"("Remote"=TRUE, "error in (no error)"=w331, "Motor Speed RPM"=w319, "UUT"=w339, "Cluster in"=w338) -> ("error out"=w335:errorcluster)  [unwired: 6 in]
            n124 = control-ref of="Motor Speed RPM"() -> (w337:refnum<vi>)
            n125 = call "Wait_Sec.vi"("Delay Time (sec)"=10.0, "error out"=w335) -> ("error in"=w314:errorcluster)  [unwired: 2 in]
            n126 = property class="DigNum (strict)"(reference=w337, error in=w314) -> (error out=w329:errorcluster, "Value"=w330:dbl)  [unwired: 1 out]
            n127 = Number To Fractional String(number=w330, precision (6)=i16 4) -> (F-format string=w326:string)  [unwired: 2 in]
            n128 = Add(x=w319, y=w320) -> (x+y=w322:dbl)
            n129 = Subtract(x=w319, y=w320) -> (x-y=w321:dbl)
            n130 = In Range and Coerce(upper limit=w322, x=w330, lower limit=w321) -> (In Range?=w328:bool)  [unwired: 1 out]
            n131 = call "PassOrFail (SubVI).vi"("disabled index (col)"=6, "index (row)"=w311, "error in (no error)"=w329, "Boolean"=w328, "Table in"=w327) -> ("error out"=w333:errorcluster)  [unwired: 6 in]
            n132 = property class="Tbl (strict)"(reference=w327, error in=w333) -> (reference out=w323:refnum<vi>, error out=w334:errorcluster, "Value"=w324:string[][])
            n133 = Replace Array Subset(array=w324, new element=w326, index (row)=w311, index (col)=5 ("disabled index (col)")) -> (w325:string[][])
            n134 = property class="Tbl (strict)"(reference=w323, error in=w334, "Value"=w325) -> (error out=w312:errorcluster)  [unwired: 1 out]
          }
          n135 = control-ref of="UUT"() -> (w286:refnum<vi>)
          n136 = control-ref of="Config_CANAT"() -> (w287:refnum<vi>)
          n137 = call "CANSendMotorSpeed.vi"("Remote"=TRUE, "error in (no error)"=w285, "Motor Speed RPM"=u16 0, "UUT"=w286, "Cluster in"=w287) -> ("error out"=w282:errorcluster)  [unwired: 6 in]
          n138 = flat-sequence {
            tunnel: [w297] -> w283
            tunnel: w282 -> [w296]
            tunnel: [w296] -> w281
            frame #0 {
              n139 = call <vilib>:"High Resolution Relative Seconds.vi"() -> ("relative seconds"=w297:dbl)
            }
          }
          n140 = while {
            tunnel: w283 -> [w305]
            tunnel: w281 -> [w298]
            tunnel: [w300] -> w258
            tunnel: [w299] -> w271
            stop <- w303 stop-if-true
            n141 = control-ref of="Motor Speed RPM"() -> (w309:refnum<vi>)
            n142 = property class="DigNum (strict)"(reference=w309, error in=w298) -> (error out=w299:errorcluster, "Value"=w308:dbl)  [unwired: 1 out]
            n143 = call <vilib>:"High Resolution Relative Seconds.vi"() -> ("relative seconds"=w306:dbl)
            n144 = Subtract(x=w306, y=w305) -> (x-y=w300:dbl)
            n145 = Greater Or Equal?(x=w300, y=50.0) -> (x >= y?=w301:bool)
            n146 = Less Or Equal?(x=w308, y=0.0) -> (x <= y?=w302:bool)
            n147 = Or(x=w302, y=w301) -> (x .or. y?=w303:bool)
          }
          n148 = call "Table_ScrollaBarMarvin.vi"("error in"=w271, "Line to focus"=w279, "reference in"=w272) -> ("error out"=w280:errorcluster)  [unwired: 2 out]
          n149 = property class="Tbl (strict)"(reference=w272, error in=w280) -> (reference out=w257:refnum<vi>, error out=w277:errorcluster, "Value"=w276:string[][])
          n150 = Index Array(array=w276, index (col)=0 ("disabled index (col)")) -> (element=w275:string[])  [unwired: 1 in]
          n151 = call "Find_Number_Line.vi"("error in"=w277, "Test Paragraph"=w279, "Row Headers[]"=w275) -> ("error out"=w273:errorcluster, "Line number"=w274:i32)  [unwired: 1 out]
          n152 = Increment(x=w274) -> (x+1=w259:i32)
          n153 = Number To Fractional String(number=w258, precision (6)=i16 4) -> (F-format string=w260:string)  [unwired: 2 in]
          n154 = Less?(x=w258, y=50.0) -> (x < y?=w262:bool)
          n155 = call "PassOrFail (SubVI).vi"("disabled index (col)"=6, "index (row)"=w259, "error in (no error)"=w273, "Boolean"=w262, "Table in"=w257) -> ("error out"=w264:errorcluster)  [unwired: 6 in]
          n156 = property class="Tbl (strict)"(reference=w257, error in=w264) -> (reference out=w269:refnum<vi>, error out=w265:errorcluster, "Value"=w268:string[][])
          n157 = Replace Array Subset(array=w268, new element=w260, index (row)=w259, index (col)=5 ("disabled index (col)")) -> (w267:string[][])
          n158 = property class="Tbl (strict)"(reference=w269, error in=w265, "Value"=w267) -> (error out=w210:errorcluster)  [unwired: 1 out]
          n159 = control-ref of="VISA resource name out"() -> (w219:refnum<vi>)
          n160 = Initialize Array(FALSE, 14 ("dimension size")) -> (w231:bool[])
          n161 = Build Array (concatenate)(w231, bool[] [FALSE, FALSE, FALSE, FALSE, FALSE, FALSE, FALSE] ("array")) -> (w232:bool[])
          n162 = Boolean Array To Number(Boolean array=w232) -> (number=w230:u32)
          n163 = property class="VISAName"(reference=w219, error in=w210) -> (error out=w218:errorcluster, "Value"=w228:refnum<visa-resource-name>)  [unwired: 1 out]
          n164 = To Unsigned Long Integer(number=w230) -> (unsigned 32bit integer=w221:u32)
          n165 = Split Number(x=w221) -> (hi(x)=w226:u16, lo(x)=w227:u16)
          n166 = Split Number(x=w227) -> (hi(x)=w225:u8, lo(x)=w224:u8)
          n167 = Split Number(x=w226) -> (hi(x)=w223:u8, lo(x)=w222:u8)
          n168 = Build Array(u8 75, u8 0 ("element"), u8 4 ("Length"), u8 2, w224, w225, w222, w223) -> (w229:u8[])
          n169 = Byte Array To String(unsigned byte array=w229) -> (string=w220:string)
          n170 = VISA Write(VISA resource name=w228, write buffer=w220, error in (no error)=w218) -> ()  [unwired: 3 out]
        }
        frame "Stop Time" {
        }
        frame "Temp Control" {
          w364 = "7.5.6" ("Test Paragraph")
          # "Venable"
          # "Deg"
          # "K15 OFF + Venable"
          # "K15 ON"
          n171 = control-ref of="Pannel User Message"() -> (w345:refnum<vi>)
          n172 = property class="Str"(reference=w345, error in=w344, "Value"="Temperature controle test") -> (error out=w343:errorcluster)  [unwired: 1 out]
          n173 = call "Table_ScrollaBarMarvin.vi"("error in"=w343, "Line to focus"=w364, "reference in"=w366) -> ("error out"=w371:errorcluster)  [unwired: 2 out]
          n174 = property class="Tbl (strict)"(reference=w366, error in=w371) -> (reference out=w341:refnum<vi>, error out=w370:errorcluster, "Value"=w369:string[][])
          n175 = Index Array(array=w369, index (col)=0 ("disabled index (col)")) -> (element=w368:string[])  [unwired: 1 in]
          n176 = control-ref of="VISA resource name out"() -> (w357:refnum<vi>)
          n177 = call "Find_Number_Line.vi"("error in"=w370, "Test Paragraph"=w364, "Row Headers[]"=w368) -> ("error out"=w365:errorcluster, "Line number"=w353:i32)  [unwired: 1 out]
          n178 = call "Table_ScrollaBarMarvin.vi"("error in"=w365, "Line to focus"=w364, "reference in"=w341) -> ("error out"=w363:errorcluster)  [unwired: 2 out]
          n179 = property class="VISAName"(reference=w357, error in=w363) -> (error out=w374:errorcluster, "Value"=w372:refnum<visa-resource-name>)  [unwired: 1 out]
          n180 = Byte Array To String(unsigned byte array=u8[] [75, 0, 4, 2, 0, 64, 2, 0] ("appended array")) -> (string=w373:string)
          n181 = VISA Write(VISA resource name=w372, write buffer=w373, error in (no error)=w374) -> (VISA resource name out=w351:refnum<visa-resource-name>, error out=w352:errorcluster)  [unwired: 1 out]
          n182 = Byte Array To String(unsigned byte array=u8[] [75, 0, 4, 2, 0, 64, 2, 0] ("appended array")) -> (string=w350:string)
          n183 = call "Wait_Sec.vi"("Delay Time (sec)"=2.0, "error out"=w352) -> ("error in"=w347:errorcluster)  [unwired: 2 in]
          n184 = VISA Write(VISA resource name=w351, write buffer=w350, error in (no error)=w347) -> (error out=w349:errorcluster)  [unwired: 2 out]
          n185 = for {
            tunnel: w357 -> [w413]
            tunnel: w349 -> [w412]
            tunnel: dbl[] [65.0, 65.0, 85.0, 85.0, 65.0] -> [w411] mode=indexing
            tunnel: dbl[] [200.0, 200.0, 400.0, 200.0, 200.0] -> [w410] mode=indexing
            tunnel: dbl[] [6000.0, 11500.0, 15100.0, 11500.0, 6000.0] -> [w409] mode=indexing
            tunnel: w353 -> [w407]
            tunnel: w341 -> [w399]
            tunnel: w341 -> [w379]
            tunnel: [w396] -> w340
            i -> [w384]
            w387 = 6 ("disabled index (col)")
            n186 = call <vilib>:"High Resolution Relative Seconds.vi"() -> ("relative seconds"=w383:dbl)
            n187 = while {
              tunnel: w413 -> [w441]
              tunnel: w411 -> [w431]
              tunnel: w410 -> [w435]
              tunnel: w409 -> [w421]
              tunnel: w412 -> [w440]
              tunnel: [w422] -> w401
              tunnel: [w429] -> w398
              tunnel: [w428] -> w397
              tunnel: [w424] -> w385
              tunnel: [w423] -> w388
              tunnel: w384 -> [w419]
              tunnel: w383 -> [w417]
              i -> [w427]
              stop <- w425 stop-if-true
              w442 = 10.0 ("y")
              n188 = case shown="4" w419 {
                tunnel: w431 -> [w468 w471 w474 w477 w480]
                tunnel: [w467 w470 w473 w476 w479] -> w430
                tunnel: w427 -> [w466 w469 w472 w475 w478]
                frame 0, Default {
                  n189 = Add(x=w468, y=w466) -> (x+y=w467:dbl)
                }
                frame 1 {
                  n190 = Add(x=w471, y=w469) -> (x+y=w470:dbl)
                }
                frame 2 {
                  n191 = Add(x=w474, y=w472) -> (x+y=w473:dbl)
                }
                frame 3 {
                  n192 = Subtract(x=w477, y=w475) -> (x-y=w476:dbl)
                }
                frame 4 {
                  n193 = Subtract(x=w480, y=w478) -> (x-y=w479:dbl)
                }
              }
              n194 = call "DegToDAC (SubVI).vi"("error in (no error)"=w440, "Numeric"=w430) -> ("error out"=w445:errorcluster, "output array"=w446:u8[])  [unwired: 8 in]
              n195 = property class="VISAName"(reference=w441, error in=w445) -> (error out=w447:errorcluster, "Value"=w449:refnum<visa-resource-name>)  [unwired: 1 out]
              n196 = Equal To 0?(x=w427) -> (x = 0?=w426:bool)
              n197 = Byte Array To String(unsigned byte array=w446) -> (string=w448:string)
              n198 = control-ref of="Ambient Temperature"() -> (w450:refnum<vi>)
              n199 = VISA Write(VISA resource name=w449, write buffer=w448, error in (no error)=w447) -> (error out=w434:errorcluster)  [unwired: 2 out]
              n200 = call "Wait_Sec.vi"("Delay Time (sec)"=5.0, "error out"=w434) -> ("error in"=w433:errorcluster)  [unwired: 2 in]
              n201 = property class="DigNum (strict)"(reference=w450, error in=w433) -> (error out=w438:errorcluster, "Value"=w424:dbl)  [unwired: 1 out]
              n202 = Subtract(x=w430, y=w442) -> (x-y=w443:dbl)
              n203 = Add(x=w430, y=w442) -> (x+y=w444:dbl)
              n204 = call <vilib>:"High Resolution Relative Seconds.vi"() -> ("relative seconds"=w418:dbl)
              n205 = control-ref of="Motor Speed RPM"() -> (w439:refnum<vi>)
              n206 = Subtract(x=w418, y=w417) -> (x-y=w416:dbl)
              n207 = In Range and Coerce(upper limit=w444, x=w424, lower limit=w443) -> (In Range?=w423:bool)  [unwired: 1 out]
              n208 = Greater Or Equal?(x=w416, y=59.0) -> (x >= y?=w414:bool)
              n209 = property class="DigNum (strict)"(reference=w439, error in=w438) -> (error out=w429:errorcluster, "Value"=w422:dbl)  [unwired: 1 out]
              n210 = case shown="0, Default" w419 {
                tunnel: w422 -> [w453 w456 w459 w462 w465]
                tunnel: w421 -> [w452 w455 w458 w461 w464]
                tunnel: [w451 w454 w457 w460 w463] -> w420
                frame 0, Default {
                  n211 = Less Or Equal?(x=w453, y=w452) -> (x <= y?=w451:bool)
                }
                frame 1 {
                  n212 = Less Or Equal?(x=w456, y=w455) -> (x <= y?=w454:bool)
                }
                frame 2 {
                  n213 = Less Or Equal?(x=w459, y=w458) -> (x <= y?=w457:bool)
                }
                frame 3 {
                  n214 = Greater Or Equal?(x=w462, y=w461) -> (x >= y?=w460:bool)
                }
                frame 4 {
                  n215 = Greater Or Equal?(x=w465, y=w464) -> (x >= y?=w463:bool)
                }
              }
              n216 = Add(x=w421, y=w435) -> (x+y=w436:dbl)
              n217 = Subtract(x=w421, y=w435) -> (x-y=w437:dbl)
              n218 = In Range and Coerce(upper limit=w436, x=w422, lower limit=w437) -> (In Range?=w428:bool)  [unwired: 1 out]
              n219 = Compound Arithmetic op=OR(w414, w420, w426) -> (w425:bool)
            }
            n220 = Multiply(x=2, y=w384) -> (x*y=w408:i32)
            n221 = Increment(x=w407) -> (x+1=w389:i32)
            n222 = Add(x=w389, y=w408) -> (x+y=w391:i32)
            n223 = call "PassOrFail (SubVI).vi"("disabled index (col)"=w387, "index (row)"=w391, "error in (no error)"=w398, "Boolean"=w397, "Table in"=w379) -> ("error out"=w404:errorcluster)  [unwired: 6 in]
            n224 = property class="Tbl (strict)"(reference=w399, error in=w404) -> (reference out=w403:refnum<vi>, error out=w381:errorcluster, "Value"=w406:string[][])
            n225 = Number To Fractional String(number=w401, precision (6)=i16 4) -> (F-format string=w405:string)  [unwired: 2 in]
            n226 = Replace Array Subset(array=w406, new element=w405, index (row)=w391, index (col)=5 ("disabled index (col)")) -> (w382:string[][])
            n227 = Increment(x=w391) -> (x+1=w386:i32)
            n228 = property class="Tbl (strict)"(reference=w379, error in=w381, "Value"=w382) -> (reference out=w377:refnum<vi>, error out=w380:errorcluster)
            n229 = call "PassOrFail (SubVI).vi"("disabled index (col)"=w387, "index (row)"=w386, "error in (no error)"=w380, "Boolean"=w388, "Table in"=w379) -> ("error out"=w378:errorcluster)  [unwired: 6 in]
            n230 = Number To Fractional String(number=w385, precision (6)=i16 4) -> (F-format string=w393:string)  [unwired: 2 in]
            n231 = property class="Tbl (strict)"(reference=w377, error in=w378) -> (error out=w375:errorcluster, "Value"=w376:string[][])  [unwired: 1 out]
            n232 = Replace Array Subset(array=w376, new element=w393, index (row)=w386, index (col)=5 ("disabled index (col)")) -> (w392:string[][])
            n233 = property class="Tbl (strict)"(reference=w403, error in=w375, "Value"=w392) -> (error out=w396:errorcluster)  [unwired: 1 out]
          }
          n234 = property class="VISAName"(reference=w357, error in=w340) -> (error out=w359:errorcluster, "Value"=w361:refnum<visa-resource-name>)  [unwired: 1 out]
          n235 = Byte Array To String(unsigned byte array=u8[] [75, 0, 4, 2, 0, 0, 0, 0] ("appended array")) -> (string=w360:string)
          n236 = VISA Write(VISA resource name=w361, write buffer=w360, error in (no error)=w359) -> ()  [unwired: 3 out]
        }
        frame "Burn in" {
          w524 = 13.0 ("y")
          w523 = 25.0 ("x")
          w519 = 2 ("disabled index (col)")
          w542 = 5.0 ("y")
          w543 = 50.0 ("x")
          w530 = 6 ("disabled index (col)")
          w551 = 400.0 ("y")
          w550 = 15100.0 ("x")
          w588 = "7.5.7" ("Test Paragraph")
          # "Get Current by ADC (2)"
          # "90Deg"
          # "Venable"
          # "K15 + Venable + 90deg OFF"
          # "K15 ON"
          n237 = property on="Stop Burn-in" class="Bool"(error in=w507, "Visible"=TRUE) -> (error out=w506:errorcluster)  [unwired: 1 in, 1 out]
          n238 = control-ref of="Pannel User Message"() -> (w574:refnum<vi>)
          n239 = property class="Str"(reference=w574, error in=w506, "Value"="Burn-in test") -> (error out=w573:errorcluster)  [unwired: 1 out]
          n240 = call "Table_ScrollaBarMarvin.vi"("error in"=w573, "Line to focus"=w588, "reference in"=w502) -> ("error out"=w594:errorcluster)  [unwired: 2 out]
          n241 = property class="Tbl (strict)"(reference=w502, error in=w594) -> (reference out=w494:refnum<vi>, error out=w593:errorcluster, "Value"=w592:string[][])
          n242 = Index Array(array=w592, index (col)=0 ("disabled index (col)")) -> (element=w591:string[])  [unwired: 1 in]
          n243 = control-ref of="VISA resource name out"() -> (w581:refnum<vi>)
          n244 = call "Find_Number_Line.vi"("error in"=w593, "Test Paragraph"=w588, "Row Headers[]"=w591) -> ("error out"=w589:errorcluster, "Line number"=w545:i32)  [unwired: 1 out]
          n245 = call "Table_ScrollaBarMarvin.vi"("error in"=w589, "Line to focus"=w588, "reference in"=w494) -> ("error out"=w587:errorcluster)  [unwired: 2 out]
          n246 = property class="VISAName"(reference=w581, error in=w587) -> (error out=w597:errorcluster, "Value"=w595:refnum<visa-resource-name>)  [unwired: 1 out]
          n247 = Increment(x=w545) -> (x+1=w531:i32)
          n248 = Byte Array To String(unsigned byte array=u8[] [75, 0, 4, 2, 0, 64, 2, 0] ("appended array")) -> (string=w596:string)
          n249 = VISA Write(VISA resource name=w595, write buffer=w596, error in (no error)=w597) -> (VISA resource name out=w579:refnum<visa-resource-name>, error out=w580:errorcluster)  [unwired: 1 out]
          n250 = Byte Array To String(unsigned byte array=u8[] [75, 0, 4, 2, 0, 64, 2, 0] ("appended array")) -> (string=w578:string)
          n251 = call "Wait_Sec.vi"("Delay Time (sec)"=2.0, "error out"=w580) -> ("error in"=w576:errorcluster)  [unwired: 2 in]
          n252 = VISA Write(VISA resource name=w579, write buffer=w578, error in (no error)=w576) -> (VISA resource name out=w567:refnum<visa-resource-name>, error out=w570:errorcluster)  [unwired: 1 out]
          n253 = call "Wait_Sec.vi"("Delay Time (sec)"=2.0, "error out"=w570) -> ("error in"=w568:errorcluster)  [unwired: 2 in]
          n254 = Byte Array To String(unsigned byte array=u8[] [75, 0, 4, 2, 0, 68, 2, 0] ("appended array")) -> (string=w569:string)
          n255 = VISA Write(VISA resource name=w567, write buffer=w569, error in (no error)=w568) -> (VISA resource name out=w560:refnum<visa-resource-name>, error out=w561:errorcluster)  [unwired: 1 out]
          n256 = call "Wait_Sec.vi"("Delay Time (sec)"=5.0, "error out"=w561) -> ("error in"=w564:errorcluster)  [unwired: 2 in]
          n257 = Byte Array To String(unsigned byte array=u8[] [75, 0, 4, 17, 0, 0, 0, 0] ("appended array")) -> (string=w563:string)
          n258 = flat-sequence {
            tunnel: w557 -> [w641]
            tunnel: [w641] -> w556
            tunnel: [w640] -> w555
            frame #0 {
              n259 = call <vilib>:"High Resolution Relative Seconds.vi"() -> ("relative seconds"=w640:dbl)
            }
          }
          n260 = VISA Write(VISA resource name=w560, write buffer=w563, error in (no error)=w564) -> (VISA resource name out=w558:refnum<visa-resource-name>, error out=w557:errorcluster)  [unwired: 1 out]
          n261 = while {
            tunnel: w558 -> [w653]
            tunnel: w556 -> [w652]
            tunnel: [w651] -> _
            tunnel: [w650] -> w554
            tunnel: w555 -> [w646]
            tunnel: [w642] -> w539
            stop <- w649 stop-if-true
            n262 = VISA Read(VISA resource name=w653, byte count=u32 1, error in (no error)=w652) -> (VISA resource name out=w655:refnum<visa-resource-name>, read buffer=w656:string, error out=w654:errorcluster)  [unwired: 1 out]
            n263 = String To Byte Array(string=w656) -> (unsigned byte array=w659:u8[])
            n264 = call <vilib>:"High Resolution Relative Seconds.vi"() -> ("relative seconds"=w647:dbl)
            n265 = Index Array(array=w659, index=0) -> (element=w657:u8)
            n266 = Subtract(x=w647, y=w646) -> (x-y=w645:dbl)
            n267 = case shown="75" w657 {
              tunnel: [w664 w668] -> w650
              tunnel: w655 -> [w663 w677]
              tunnel: w654 -> [w664 w676]
              tunnel: [w663 w669] -> w651
              tunnel: [FALSE w666] -> w648
              tunnel: [u32 9999 w665] -> w642
              frame 0, Default {
              }
              frame 75 {
                n268 = VISA Read(VISA resource name=w677, byte count=u32 3, error in (no error)=w676) -> (VISA resource name out=w672:refnum<visa-resource-name>, read buffer=w680:string, error out=w671:errorcluster)  [unwired: 1 out]
                n269 = String To Byte Array(string=w680) -> (unsigned byte array=w670:u8[])
                n270 = Index Array(array=w670, index #1=0 ("index")) -> (element #1=w675:u8, element #2=w673:u8)  [unwired: 2 in, 1 out]
                n271 = Equal?(x=u8 0, y=w675) -> (x = y?=w674:bool)
                n272 = case shown="True" w674 {
                  tunnel: [w683 w691] -> w668
                  tunnel: w673 -> [_ w698]
                  tunnel: w672 -> [w684 w697]
                  tunnel: w671 -> [w683 w696]
                  tunnel: w670 -> [_ w695]
                  tunnel: [w684 w693] -> w669
                  tunnel: [FALSE TRUE] -> w666
                  tunnel: [u32 9999 w685] -> w665
                  frame False {
                  }
                  frame True {
                    n273 = VISA Read(VISA resource name=w697, byte count=w698, error in (no error)=w696) -> (VISA resource name out=w693:refnum<visa-resource-name>, read buffer=w692:string, error out=w691:errorcluster)  [unwired: 1 out]
                    n274 = String To Byte Array(string=w692) -> (unsigned byte array=w694:u8[])
                    n275 = Insert Into Array(array=w695, index=0, new element=w694) -> (w686:u8[])
                    n276 = Index Array(array=w686, index #1=0 ("index")) -> (element #3=w687:u8)  [unwired: 2 in, 2 out]
                    n277 = case shown="15..19" w687 {
                      tunnel: w686 -> [_ w707]
                      tunnel: [u32 9999 w700] -> w685
                      frame 0, Default {
                      }
                      frame 15..19 {
                        n278 = Index Array(array=w707, index #1=3 ("index")) -> (element #1=w706:u8, element #2=w705:u8, element #3=w704:u8, element #4=w703:u8)  [unwired: 3 in]
                        n279 = Join Numbers(hi=w705, lo=w706) -> ((hi.lo)=w702:u16)
                        n280 = Join Numbers(hi=w703, lo=w704) -> ((hi.lo)=w701:u16)
                        n281 = Join Numbers(hi=w701, lo=w702) -> ((hi.lo)=w700:u32)
                      }
                    }
                  }
                }
              }
            }
            n282 = Greater Or Equal?(x=w645, y=10.0) -> (x >= y?=w643:bool)
            n283 = Or(x=w648, y=w643) -> (x .or. y?=w649:bool)
          }
          n284 = control-ref of="Motor Speed RPM"() -> (w565:refnum<vi>)
          n285 = Add(x=w543, y=w542) -> (x+y=w541:dbl)
          n286 = Subtract(x=w543, y=w542) -> (x-y=w540:dbl)
          n287 = In Range and Coerce(upper limit=w541, x=w539, lower limit=w540) -> (In Range?=w538:bool)  [unwired: 1 out]
          n288 = property class="DigNum (strict)"(reference=w565, error in=w554) -> (error out=w521:errorcluster, "Value"=w510:dbl)  [unwired: 1 out]
          n289 = Number To Fractional String(number=w510, precision (6)=i16 4) -> (F-format string=w535:string)  [unwired: 2 in]
          n290 = Add(x=w550, y=w551) -> (x+y=w552:dbl)
          n291 = Subtract(x=w550, y=w551) -> (x-y=w553:dbl)
          n292 = In Range and Coerce(upper limit=w552, x=w510, lower limit=w553) -> (In Range?=w528:bool)  [unwired: 1 out]
          n293 = Increment(x=w531) -> (x+1=w529:i32)
          n294 = control-ref of="Ambient Temperature"() -> (w525:refnum<vi>)
          n295 = property class="DigNum (strict)"(reference=w525, error in=w521) -> (error out=w522:errorcluster, "Value"=w515:dbl)  [unwired: 1 out]
          n296 = Add(x=w515, y=25.0) -> (x+y=w508:dbl)
          n297 = Number To Fractional String(number=w508, precision (6)=i16 0) -> (F-format string=w513:string)  [unwired: 2 in]
          n298 = Concatenate Strings("< " ("string"), w513) -> (w512:string)
          n299 = Add(x=w523, y=w524) -> (x+y=w526:dbl)
          n300 = Subtract(x=w523, y=w524) -> (x-y=w527:dbl)
          n301 = Number To Fractional String(number=w515, precision (6)=i16 4) -> (F-format string=w534:string)  [unwired: 2 in]
          n302 = Increment(x=w529) -> (x+1=w500:i32)
          n303 = Increment(x=w500) -> (x+1=w518:i32)
          n304 = Increment(x=w518) -> (x+1=w517:i32)
          n305 = Increment(x=w517) -> (x+1=w499:i32)
          n306 = In Range and Coerce(upper limit=w526, x=w515, lower limit=w527) -> (In Range?=w520:bool)  [unwired: 1 out]
          n307 = property class="Tbl (strict)"(reference=w494, error in=w522) -> (reference out=w544:refnum<vi>, error out=w489:errorcluster, "Value"=w549:string[][])
          n308 = Number To Fractional String(number=w539, precision (6)=i16 4) -> (F-format string=w548:string)  [unwired: 2 in]
          n309 = Replace Array Subset(array=w549, new element=w548, index (row)=w531, index (col)=5 ("disabled index (col)")) -> (w497:string[][])
          n310 = property class="Tbl (strict)"(reference=w494, error in=w489, "Value"=w497) -> (reference out=w496:refnum<vi>, error out=w488:errorcluster)
          n311 = call "PassOrFail (SubVI).vi"("disabled index (col)"=w530, "index (row)"=w531, "error in (no error)"=w488, "Boolean"=w538, "Table in"=w544) -> ("error out"=w487:errorcluster)  [unwired: 6 in]
          n312 = property class="Tbl (strict)"(reference=w496, error in=w487) -> (reference out=w492:refnum<vi>, error out=w486:errorcluster, "Value"=w495:string[][])
          n313 = Replace Array Subset(array=w495, new element=w535, index (row)=w529, index (col)=5 ("disabled index (col)")) -> (w493:string[][])
          n314 = property class="Tbl (strict)"(reference=w492, error in=w486, "Value"=w493) -> (reference out=w491:refnum<vi>, error out=w485:errorcluster)
          n315 = call "PassOrFail (SubVI).vi"("disabled index (col)"=w530, "index (row)"=w529, "error in (no error)"=w485, "Boolean"=w528, "Table in"=w494) -> ("error out"=w484:errorcluster)  [unwired: 6 in]
          n316 = property class="Tbl (strict)"(reference=w491, error in=w484) -> (error out=w483:errorcluster, "Value"=w490:string[][])  [unwired: 1 out]
          n317 = Replace Array Subset(array=w490, new element #1=w534, index (row) #1=w500, index (col) #1=5 ("disabled index (col)"), new element #2=w512, index (row) #2=w518, index (col) #2=w519, new element #3=w512, index (row) #3=w517, index (col) #3=w519, new element #4=w512, index (row) #4=w499, index (col) #4=w519) -> (w532:string[][])
          n318 = property class="Tbl (strict)"(reference=w494, error in=w483, "Value"=w532) -> (error out=w482:errorcluster)  [unwired: 1 out]
          n319 = call "PassOrFail (SubVI).vi"("disabled index (col)"=w530, "index (row)"=w500, "error in (no error)"=w482, "Boolean"=w520, "Table in"=w494) -> ("error out"=w481:errorcluster)  [unwired: 6 in]
          n320 = for {
            tunnel: w481 -> [w622]
            tunnel: dbl[] [600.0, 1200.0, 1800.0] -> [w619] mode=indexing
            tunnel: w508 -> [w616]
            tunnel: w500 -> [w613]
            tunnel: w502 -> [w607]
            tunnel: [w598] -> w501
            i -> [w612]
            n321 = Increment(x=w612) -> (x+1=w611:i32)
            n322 = flat-sequence {
              tunnel: [w638] -> _
              tunnel: [w638] -> w621
              tunnel: [w639] -> w620
              tunnel: w622 -> [w638]
              frame #0 {
                n323 = call <vilib>:"High Resolution Relative Seconds.vi"() -> ("relative seconds"=w639:dbl)
              }
            }
            n324 = Add(x=w613, y=w611) -> (x+y=w605:i32)
            n325 = while {
              tunnel: w621 -> [w633]
              tunnel: w620 -> [w636]
              tunnel: w619 -> [w627]
              tunnel: [w624] -> w617
              stop <- w623 stop-if-true
              n326 = call <vilib>:"High Resolution Relative Seconds.vi"() -> ("relative seconds"=w637:dbl)
              n327 = Subtract(x=w637, y=w636) -> (x-y=w626:dbl)
              n328 = control-ref of="Pannel User Message"() -> (w632:refnum<vi>)
              n329 = Greater Or Equal?(x=w626, y=w627) -> (x >= y?=w635:bool)
              n330 = Or(x="Stop Burn-in", y=w635) -> (x .or. y?=w623:bool)
              n331 = Subtract(x=w627, y=w626) -> (x-y=w628:dbl)
              n332 = Number To Fractional String(number=w628, precision (6)=i16 4) -> (F-format string=w629:string)  [unwired: 2 in]
              n333 = Concatenate Strings("Remained Time: " ("string"), w629) -> (w625:string)
              n334 = property class="Str"(reference=w632, error in=w633, "Value"=w625) -> (error out=w624:errorcluster)  [unwired: 1 out]
            }
            n335 = control-ref of="Power transistor Heat sink Temp."() -> (w618:refnum<vi>)
            n336 = property class="DigNum (strict)"(reference=w618, error in=w617) -> (error out=w608:errorcluster, "Value"=w609:dbl)  [unwired: 1 out]
            n337 = Less Or Equal?(x=w609, y=w616) -> (x <= y?=w602:bool)
            n338 = property class="Tbl (strict)"(reference=w607, error in=w608) -> (reference out=w601:refnum<vi>, error out=w600:errorcluster, "Value"=w604:string[][])
            n339 = Number To Fractional String(number=w609, precision (6)=i16 4) -> (F-format string=w610:string)  [unwired: 2 in]
            n340 = Replace Array Subset(array=w604, new element=w610, index (row)=w605, index (col)=5 ("disabled index (col)")) -> (w603:string[][])
            n341 = property class="Tbl (strict)"(reference=w601, error in=w600, "Value"=w603) -> (error out=w599:errorcluster)  [unwired: 1 out]
            n342 = call "PassOrFail (SubVI).vi"("disabled index (col)"=6, "index (row)"=w605, "error in (no error)"=w599, "Boolean"=w602, "Table in"=w601) -> ("error out"=w598:errorcluster)  [unwired: 6 in]
          }
          n343 = property on="Stop Burn-in" class="Bool"(error in=w501, "Visible"=FALSE) -> (error out=w503:errorcluster)  [unwired: 1 in, 1 out]
          n344 = property class="VISAName"(reference=w581, error in=w503) -> (error out=w583:errorcluster, "Value"=w585:refnum<visa-resource-name>)  [unwired: 1 out]
          n345 = Byte Array To String(unsigned byte array=u8[] [75, 0, 4, 2, 0, 0, 0, 0] ("appended array")) -> (string=w584:string)
          n346 = VISA Write(VISA resource name=w585, write buffer=w584, error in (no error)=w583) -> ()  [unwired: 3 out]
        }
        frame "Visual Inspec" {
          n347 = call "VisualInspection.vi"("error in (no error)"=w710, "TableRef"=w709) -> ()  [unwired: 9 in, 1 out]
        }
        frame "Temp Sens Cal" {
          w730 = "7.5.5" ("Test Paragraph")
          n348 = control-ref of="Pannel User Message"() -> (w714:refnum<vi>)
          n349 = property class="Str"(reference=w714, error in=w713, "Value"="Temperature sensor calibration test") -> (error out=w712:errorcluster)  [unwired: 1 out]
          n350 = call "Table_ScrollaBarMarvin.vi"("error in"=w712, "Line to focus"=w730, "reference in"=w726) -> ("error out"=w729:errorcluster)  [unwired: 2 out]
          n351 = property class="Tbl (strict)"(reference=w726, error in=w729) -> (error out=w732:errorcluster, "Value"=w733:string[][])  [unwired: 1 out]
          n352 = Concatenate Strings("EP=1\r\nAO" ("string"), "[", "1" ("string"), "]=0", "\r\n" ("write buffer")) -> (w720:string)
          n353 = Index Array(array=w733, index (col)=0 ("disabled index (col)")) -> (element=w734:string[])  [unwired: 1 in]
          n354 = call "Find_Number_Line.vi"("error in"=w732, "Test Paragraph"=w730, "Row Headers[]"=w734) -> ("error out"=w728:errorcluster, "Line number"=w725:i32)  [unwired: 1 out]
          n355 = property on="Status" class="Bool (strict)"(error in=w728) -> (error out=w719:errorcluster, "Value"=w727:bool)  [unwired: 1 in, 1 out]
          n356 = call "SerialMarvinMod.vi"("error in (no error)"=w719, "Clear Log"=FALSE, "write buffer"=w720, "VISA resource name"=w717) -> ("error out"=w718:errorcluster)  [unwired: 6 in, 1 out]
          n357 = case shown="True" w727 {
            selector: w727 -> [w739 _]
            tunnel: w718 -> [w741 w774]
            tunnel: w726 -> [w738 w749]
            tunnel: w725 -> [w737 w748]
            tunnel: w717 -> [_ w753]
            frame False {
              n358 = flat-sequence {
                tunnel: w741 -> [w742]
                tunnel: [w742] -> w740
                frame #0 {
                  n359 = One Button Dialog(message="Please establish RS connection.") -> ()  [unwired: 1 in, 1 out]
                }
              }
              n360 = Increment(x=w737) -> (x+1=w736:i32)
              n361 = call "PassOrFail (SubVI).vi"("disabled index (col)"=6, "index (row)"=w736, "error in (no error)"=w740, "Boolean"=w739, "Table in"=w738) -> ()  [unwired: 6 in, 1 out]
            }
            frame True {
              n362 = for {
                tunnel: u32[] [64, 512, 2048, 8192] -> [w814] mode=indexing
                tunnel: w753 -> [w809]
                tunnel: dbl[] [0.59774, 0.65238, 0.68545, 0.71584] -> [w807] mode=indexing
                tunnel: [w798] -> w795 mode=indexing
                tunnel: [w806] -> w789
                tunnel: w774 -> [w804]
                tunnel: [w802] -> w755
                tunnel: [w801] -> w744 mode=indexing
                n363 = control-ref of="VISA resource name out"() -> (w811:refnum<vi>)
                n364 = To Unsigned Long Integer(number=w814) -> (unsigned 32bit integer=w816:u32)
                n365 = Split Number(x=w816) -> (hi(x)=w821:u16, lo(x)=w822:u16)
                n366 = property class="VISAName"(reference=w811, error in=w804) -> (error out=w805:errorcluster, "Value"=w802:refnum<visa-resource-name>)  [unwired: 1 out]
                n367 = Split Number(x=w822) -> (hi(x)=w820:u8, lo(x)=w819:u8)
                n368 = Split Number(x=w821) -> (hi(x)=w818:u8, lo(x)=w817:u8)
                n369 = Build Array(u8 75, u8 0 ("element"), u8 4 ("Length"), u8 2, w819, w820, w817, w818) -> (w813:u8[])
                n370 = Byte Array To String(unsigned byte array=w813) -> (string=w812:string)
                n371 = VISA Write(VISA resource name=w802, write buffer=w812, error in (no error)=w805) -> (error out=w808:errorcluster)  [unwired: 2 out]
                n372 = Concatenate Strings("TA" ("string"), "[", "5" ("string"), "]", "\r\n" ("write buffer")) -> (w826:string)
                n373 = call "Wait_Sec.vi"("Delay Time (sec)"=2.0, "error out"=w808) -> ("error in"=w800:errorcluster)  [unwired: 2 in]
                n374 = call "SerialMarvinMod.vi"("error in (no error)"=w800, "Clear Log"=FALSE, "write buffer"=w826, "VISA resource name"=w809) -> ("error out"=w806:errorcluster, "read buffer"=w803:string)  [unwired: 6 in]
                n375 = Fract/Exp String To Number(string=w803) -> (number=w801:dbl)  [unwired: 3 in, 1 out]
                n376 = Subtract(x=w801, y=w807) -> (x-y=w798:dbl)
              }
              "Array 2" <- w744
              n377 = Add Array Elements(numeric array=w795) -> (sum=w794:dbl)
              n378 = Divide(x=w794, y=4.0) -> (x/y=w767:dbl)
              n379 = In Range and Coerce(upper limit=0.1, x=w767, lower limit=-0.1) -> (In Range?=w745:bool)  [unwired: 1 out]
              n380 = Number To Fractional String(number=w767, precision (6)=i16 4) -> (F-format string=w750:string)  [unwired: 2 in]
              n381 = Increment(x=w748) -> (x+1=w765:i32)
              n382 = call "PassOrFail (SubVI).vi"("disabled index (col)"=6, "index (row)"=w765, "error in (no error)"=w789, "Boolean"=w745, "Table in"=w749) -> ("error out"=w769:errorcluster)  [unwired: 6 in]
              n383 = To Unsigned Long Integer(number=u32 0) -> (unsigned 32bit integer=w777:u32)
              n384 = property class="Tbl (strict)"(reference=w749, error in=w769) -> (reference out=w773:refnum<vi>, error out=w772:errorcluster, "Value"=w770:string[][])
              n385 = Split Number(x=w777) -> (hi(x)=w783:u16, lo(x)=w784:u16)
              n386 = Split Number(x=w784) -> (hi(x)=w782:u8, lo(x)=w781:u8)
              n387 = Split Number(x=w783) -> (hi(x)=w780:u8, lo(x)=w779:u8)
              n388 = Replace Array Subset(array=w770, new element=w750, index (row)=w765, index (col)=5 ("disabled index (col)")) -> (w771:string[][])
              n389 = property class="Tbl (strict)"(reference=w773, error in=w772, "Value"=w771) -> (error out=w768:errorcluster)  [unwired: 1 out]
              n390 = Build Array(u8 75, u8 0 ("element"), u8 4 ("Length"), u8 2, w781, w782, w779, w780) -> (w775:u8[])
              n391 = Byte Array To String(unsigned byte array=w775) -> (string=w788:string)
              n392 = VISA Write(VISA resource name=w755, write buffer=w788, error in (no error)=w768) -> (error out=w756:errorcluster)  [unwired: 2 out]
              n393 = Concatenate Strings("EP=1\r\nAO" ("string"), "[", "1" ("string"), "]=", w750, "\r\n" ("write buffer")) -> (w759:string)
              n394 = call "SerialMarvinMod.vi"("error in (no error)"=w756, "Clear Log"=FALSE, "write buffer"=w759, "VISA resource name"=w753) -> ("error out"=w754:errorcluster)  [unwired: 6 in, 1 out]
              n395 = call "SerialMarvinMod.vi"("error in (no error)"=w754, "write buffer"="AO[1]\r\n", "VISA resource name"=w753) -> ("error out"=w746:errorcluster, "read buffer"=w751:string)  [unwired: 7 in]
              n396 = Equal?(x=w750, y=w751) -> ()  [unwired: 1 out]
              n397 = call "PassOrFail (SubVI).vi"("disabled index (col)"=6, "index (row)"=w748, "error in (no error)"=w746, "Boolean"=w745, "Table in"=w749) -> ()  [unwired: 6 in, 1 out]
            }
          }
        }
        frame "Auxiliary" {
          w854 = "8" ("Test Paragraph")
          # "K20 OFF"
          # "K20 ON"
          # "Venable"
          # "OFF"
          n398 = control-ref of="Pannel User Message"() -> (w843:refnum<vi>)
          n399 = property class="Str"(reference=w843, error in=w838, "Value"="Auxiliary test") -> (error out=w842:errorcluster)  [unwired: 1 out]
          n400 = call "Table_ScrollaBarMarvin.vi"("error in"=w842, "Line to focus"=w854, "reference in"=w839) -> ("error out"=w860:errorcluster)  [unwired: 2 out]
          n401 = property class="Tbl (strict)"(reference=w839, error in=w860) -> (reference out=w833:refnum<vi>, error out=w859:errorcluster, "Value"=w858:string[][])
          n402 = Index Array(array=w858, index (col)=0 ("disabled index (col)")) -> (element=w857:string[])  [unwired: 1 in]
          n403 = control-ref of="VISA resource name out"() -> (w848:refnum<vi>)
          n404 = call "Find_Number_Line.vi"("error in"=w859, "Test Paragraph"=w854, "Row Headers[]"=w857) -> ("error out"=w855:errorcluster, "Line number"=w840:i32)  [unwired: 1 out]
          n405 = call "Table_ScrollaBarMarvin.vi"("error in"=w855, "Line to focus"=w854, "reference in"=w833) -> ("error out"=w853:errorcluster)  [unwired: 2 out]
          n406 = property class="VISAName"(reference=w848, error in=w853) -> (error out=w863:errorcluster, "Value"=w861:refnum<visa-resource-name>)  [unwired: 1 out]
          n407 = Byte Array To String(unsigned byte array=u8[] [75, 0, 4, 2, 0, 0, 2, 0] ("appended array")) -> (string=w862:string)
          n408 = VISA Write(VISA resource name=w861, write buffer=w862, error in (no error)=w863) -> (VISA resource name out=w846:refnum<visa-resource-name>, error out=w847:errorcluster)  [unwired: 1 out]
          n409 = Build Array(u8[] [75, 0, 4, 2, 0, 0, 10, 0] ("appended array"), u8[] [75, 0, 4, 2, 0, 0, 2, 0] ("appended array")) -> (w834:u8[][])
          n410 = call "Wait_Sec.vi"("Delay Time (sec)"=2.0, "error out"=w847) -> ("error in"=w845:errorcluster)  [unwired: 2 in]
          n411 = for {
            tunnel: w846 -> [w905]
            tunnel: w845 -> [w903]
            tunnel: w834 -> [w898] mode=indexing
            tunnel: w833 -> [w878]
            tunnel: w840 -> [w884]
            tunnel: [w879] -> w832
            i -> [w882]
            w889 = 6 ("disabled index (col)")
            n412 = Byte Array To String(unsigned byte array=w898) -> (string=w904:string)
            n413 = flat-sequence {
              tunnel: w897 -> [w996]
              tunnel: [w996] -> w896
              tunnel: [w995] -> w900
              frame #0 {
                n414 = call <vilib>:"High Resolution Relative Seconds.vi"() -> ("relative seconds"=w995:dbl)
              }
            }
            n415 = VISA Write(VISA resource name=w905, write buffer=w904, error in (no error)=w903) -> (VISA resource name out=w899:refnum<visa-resource-name>, error out=w902:errorcluster)  [unwired: 1 out]
            n416 = call "Wait_Sec.vi"("Delay Time (sec)"=5.0, "error out"=w902) -> ("error in"=w897:errorcluster)  [unwired: 2 in]
            n417 = while {
              tunnel: w900 -> [w933]
              tunnel: w899 -> [w932]
              tunnel: w896 -> [w914]
              tunnel: [w912] -> w877
              tunnel: [w911] -> _
              tunnel: [w907] -> w880
              tunnel: [w910] -> w883
              tunnel: w882 -> [w909]
              tunnel: [w908] -> w881
              tunnel: [w906] -> w876
              stop <- w913 stop-if-true
              # "Get Current by ADC (2)"
              n418 = Byte Array To String(unsigned byte array=u8[] [75, 0, 4, 17, 0, 0, 0, 0] ("appended array")) -> (string=w931:string)
              n419 = VISA Write(VISA resource name=w932, write buffer=w931, error in (no error)=w914) -> (VISA resource name out=w917:refnum<visa-resource-name>, error out=w918:errorcluster)  [unwired: 1 out]
              n420 = VISA Read(VISA resource name=w917, byte count=u32 1, error in (no error)=w918) -> (VISA resource name out=w925:refnum<visa-resource-name>, read buffer=w926:string, error out=w924:errorcluster)  [unwired: 1 out]
              n421 = call <vilib>:"High Resolution Relative Seconds.vi"() -> ("relative seconds"=w922:dbl)
              n422 = String To Byte Array(string=w926) -> (unsigned byte array=w929:u8[])
              n423 = Index Array(array=w929, index=0) -> (element=w927:u8)
              n424 = Subtract(x=w922, y=w933) -> (x-y=w921:dbl)
              n425 = case shown="75" w927 {
                tunnel: [w950 w954] -> w915
                tunnel: w925 -> [w949 w963]
                tunnel: w924 -> [w950 w962]
                tunnel: [w949 w955] -> w911
                tunnel: [FALSE w952] -> w923
                tunnel: [u32 9999 w951] -> w907
                frame 0, Default {
                }
                frame 75 {
                  n426 = VISA Read(VISA resource name=w963, byte count=u32 3, error in (no error)=w962) -> (VISA resource name out=w958:refnum<visa-resource-name>, read buffer=w966:string, error out=w957:errorcluster)  [unwired: 1 out]
                  n427 = String To Byte Array(string=w966) -> (unsigned byte array=w956:u8[])
                  n428 = Index Array(array=w956, index #1=0 ("index")) -> (element #1=w961:u8, element #2=w959:u8)  [unwired: 2 in, 1 out]
                  n429 = Equal?(x=u8 0, y=w961) -> (x = y?=w960:bool)
                  n430 = case shown="True" w960 {
                    tunnel: [w969 w977] -> w954
                    tunnel: w959 -> [_ w984]
                    tunnel: w958 -> [w970 w983]
                    tunnel: w957 -> [w969 w982]
                    tunnel: w956 -> [_ w981]
                    tunnel: [w970 w979] -> w955
                    tunnel: [FALSE TRUE] -> w952
                    tunnel: [u32 9999 w971] -> w951
                    frame False {
                    }
                    frame True {
                      n431 = VISA Read(VISA resource name=w983, byte count=w984, error in (no error)=w982) -> (VISA resource name out=w979:refnum<visa-resource-name>, read buffer=w978:string, error out=w977:errorcluster)  [unwired: 1 out]
                      n432 = String To Byte Array(string=w978) -> (unsigned byte array=w980:u8[])
                      n433 = Insert Into Array(array=w981, index=0, new element=w980) -> (w972:u8[])
                      n434 = Index Array(array=w972, index #1=0 ("index")) -> (element #3=w973:u8)  [unwired: 2 in, 2 out]
                      n435 = case shown="15..19" w973 {
                        tunnel: w972 -> [_ w993]
                        tunnel: [u32 9999 w986] -> w971
                        frame 0, Default {
                        }
                        frame 15..19 {
                          n436 = Index Array(array=w993, index #1=3 ("index")) -> (element #1=w992:u8, element #2=w991:u8, element #3=w990:u8, element #4=w989:u8)  [unwired: 3 in]
                          n437 = Join Numbers(hi=w991, lo=w992) -> ((hi.lo)=w988:u16)
                          n438 = Join Numbers(hi=w989, lo=w990) -> ((hi.lo)=w987:u16)
                          n439 = Join Numbers(hi=w987, lo=w988) -> ((hi.lo)=w986:u32)
                        }
                      }
                    }
                  }
                }
              }
              n440 = Greater Or Equal?(x=w921, y=30.0) -> (x >= y?=w919:bool)
              n441 = control-ref of="Ambient Temperature"() -> (w916:refnum<vi>)
              n442 = property class="DigNum (strict)"(reference=w916, error in=w915) -> (error out=w912:errorcluster, "Value"=w910:dbl)  [unwired: 1 out]
              n443 = case shown="0, Default" w909 {
                tunnel: [w939 w945] -> w908
                tunnel: w910 -> [w938 w946]
                tunnel: w907 -> [w937 w943]
                tunnel: [w935 w941] -> w906
                frame 0, Default {
                  n444 = Greater?(x=w937, y=u32 2) -> (0:w935:bool)
                  n445 = Greater?(x=w938, y=63.0) -> (0:w939:bool)
                }
                frame 1 {
                  n446 = Less?(x=w943, y=u32 1) -> (x < y?=w941:bool)
                  n447 = Less Or Equal?(x=w946, y=55.0) -> (x <= y?=w945:bool)
                }
              }
              n448 = Compound Arithmetic op=OR(w908, w923, w919) -> (w913:bool)
            }
            n449 = Multiply(x=w882, y=2) -> (x*y=w873:i32)
            n450 = Increment(x=w873) -> (x+1=w874:i32)
            n451 = Add(x=w884, y=w874) -> (x+y=w875:i32)
            n452 = call "PassOrFail (SubVI).vi"("disabled index (col)"=w889, "index (row)"=w875, "error in (no error)"=w877, "Boolean"=w881, "Table in"=w878) -> ("error out"=w893:errorcluster)  [unwired: 6 in]
            n453 = property class="Tbl (strict)"(reference=w878, error in=w893) -> (reference out=w868:refnum<vi>, error out=w866:errorcluster, "Value"=w895:string[][])
            n454 = Number To Fractional String(number=w883, precision (6)=i16 4) -> (F-format string=w894:string)  [unwired: 2 in]
            n455 = Replace Array Subset(array=w895, new element=w894, index (row)=w875, index (col)=5 ("disabled index (col)")) -> (w871:string[][])
            n456 = property class="Tbl (strict)"(reference=w868, error in=w866, "Value"=w871) -> (reference out=w869:refnum<vi>, error out=w865:errorcluster)
            n457 = Increment(x=w875) -> (x+1=w890:i32)
            n458 = Number To Fractional String(number=w880, precision (6)=i16 4) -> (F-format string=w892:string)  [unwired: 2 in]
            n459 = call "PassOrFail (SubVI).vi"("disabled index (col)"=w889, "index (row)"=w890, "error in (no error)"=w865, "Boolean"=w876, "Table in"=w878) -> ("error out"=w864:errorcluster)  [unwired: 6 in]
            n460 = property class="Tbl (strict)"(reference=w869, error in=w864) -> (error out=w867:errorcluster, "Value"=w870:string[][])  [unwired: 1 out]
            n461 = Replace Array Subset(array=w870, new element=w892, index (row)=w890, index (col)=5 ("disabled index (col)")) -> (w891:string[][])
            n462 = property class="Tbl (strict)"(reference=w868, error in=w867, "Value"=w891) -> (error out=w879:errorcluster)  [unwired: 1 out]
          }
          n463 = property class="VISAName"(reference=w848, error in=w832) -> (error out=w850:errorcluster, "Value"=w852:refnum<visa-resource-name>)  [unwired: 1 out]
          n464 = Byte Array To String(unsigned byte array=u8[] [75, 0, 4, 2, 0, 0, 0, 0] ("appended array")) -> (string=w851:string)
          n465 = VISA Write(VISA resource name=w852, write buffer=w851, error in (no error)=w850) -> ()  [unwired: 3 out]
        }
      }
    }
  }
  n466 = disable-structure shown="Disabled" {
    frame Disabled {
      n467 = property class="Tbl (strict)"() -> (reference=w1011:refnum<vi>, error out=w1010:errorcluster, "Value"=w1003:string[][])  [unwired: 1 in, 1 out]
      n468 = Replace Array Subset(array=w1003, index (row)=0, index (col)=5 ("disabled index (col)")) -> (w1004:string[][], new element=w1007:string)
      n469 = Equal?(x="PASS") -> (y=w1008:string, x = y?=w998:bool)
      n470 = Select(t=u32 6618880, s=w998, f=u32 16711680) -> (s? t:f=w1002:u32)
      n471 = property class="Tbl (strict)"(reference=w1011, error in=w1010, "Active Cell"=T12 {"Row"=0, "Column"=5} ("Active Cell:Active Cell"), "Cell BG Color"=w1002) -> (error out=w1009:errorcluster)  [unwired: 1 out]
      n472 = property class="Tbl (strict)"(reference=w1011, error in=w1009, "Value"=w1004) -> ()  [unwired: 2 out]
    }
    frame Enabled {
    }
  }
  n473 = while {
    shift-right: [w1020] -> _
    shift-left: w8 -> [w1022]
    shift-right: [w1018] -> _
    shift-left: _ -> [w1019]
    shift-right: [w1015] -> _
    shift-left: _ -> [w1014]
    shift-right: [w1012] -> _
    shift-left: w4 -> [w1012]
    stop <- w1021 stop-if-true
    n474 = Dequeue Element(queue=w1022, error in (no error)=w1012) -> (queue out=w1020:refnum<queue>, element=w1013:T9, error out=w1021:errorcluster)  [unwired: 1 in, 1 out]
    n475 = for {
      tunnel: [w1143] -> w1017 mode=indexing
      tunnel: w1013 -> [w1142] mode=indexing
      tunnel: [w1141] -> w1016 mode=indexing
      n476 = Unbundle By Name(w1142) -> ("aDATA"=w1141:u8[])
      n477 = call "Array Data to Single Num in Hex.vi"("aDATA"=w1141) -> ("Numeric"=w1143:u64)  [unwired: 10 in]
    }
    n478 = Build Array (concatenate)(w1017, w1019) -> (w1018:u64[][])
    "Array" <- w1018
    n479 = for {
      tunnel: w1016 -> [w1027] mode=indexing
      tunnel: [w1025] -> w1015
      tunnel: w1014 -> [w1024]
      tunnel: w1013 -> [w1023]
      i -> [w1026]
      n480 = case shown="0, Default" w1026 {
        tunnel: w1027 -> [w1066 w1104 w1136]
        tunnel: [w1040 w1099 w1131] -> w1025
        tunnel: w1024 -> [w1041 w1099 w1131]
        tunnel: w1023 -> [w1039 _ _]
        frame 0, Default {
          # "Frame ID\n0x18E1273F"
          n481 = Index Array(array=w1066, index #1=0 ("index"), index #2=1 ("index"), index #3=2 ("index"), index #4=3 ("index"), index #5=4 ("index"), index #6=5 ("index"), index #7=6 ("index"), index #8=7 ("index")) -> (element #1=w1050:u8, element #2=w1052:u8, element #3=w1053:u8, element #4=w1057:u8, element #5=w1060:u8, element #6=w1064:u8, element #7=w1065:u8, element #8=w1063:u8)
          n482 = Number To Hexadecimal String(2:w1063) -> (0:w1077:string)  [unwired: 1 in]
          n483 = Join Numbers(hi=w1065, lo=w1064) -> ((hi.lo)=w1084:u16)
          n484 = Join Numbers(hi=w1053, lo=w1052) -> ((hi.lo)=w1054:u16)
          n485 = Number To Hexadecimal String(2:w1060) -> (0:w1061:string)  [unwired: 1 in]
          n486 = Number To Hexadecimal String(2:w1084) -> (0:w1083:string)  [unwired: 1 in]
          n487 = Number To Hexadecimal String(2:w1050) -> (0:w1051:string)  [unwired: 1 in]
          n488 = Number To Hexadecimal String(2:w1054) -> (0:w1055:string)  [unwired: 1 in]
          n489 = Number To Hexadecimal String(2:w1057) -> (0:w1058:string)  [unwired: 1 in]
          n490 = Hexadecimal String To Number(string=w1077) -> (number=w1076:u32)  [unwired: 2 in, 1 out]
          n491 = Index Array(array=w1039, index=0) -> (element=w1037:T13)
          n492 = To Double Precision Float(number=w1076) -> (double precision float=→"DC Current":dbl)
          n493 = Unbundle By Name(w1037) -> ("ID"=w1029:u32)
          n494 = Hexadecimal String To Number(string=w1061) -> (number=w1062:u32)  [unwired: 2 in, 1 out]
          n495 = Hexadecimal String To Number(string=w1083) -> (number=w1082:u32)  [unwired: 2 in, 1 out]
          n496 = Hexadecimal String To Number(string=w1051) -> (number=w1048:u32)  [unwired: 2 in, 1 out]
          n497 = Hexadecimal String To Number(string=w1055) -> (number=w1056:u32)  [unwired: 2 in, 1 out]
          n498 = Hexadecimal String To Number(string=w1058) -> (number=w1059:u32)  [unwired: 2 in, 1 out]
          n499 = To Double Precision Float(number=u32 10 ("y")) -> (double precision float=w1080:dbl)
          n500 = To Double Precision Float(number=w1082) -> (double precision float=w1079:dbl)
          n501 = To Double Precision Float(number=w1062) -> (double precision float=w1043:dbl)
          n502 = To Double Precision Float(number=w1056) -> (double precision float=w1036:dbl)
          "Motor Speed RPM" <- w1036
          n503 = To Double Precision Float(number=w1059) -> (double precision float=w1045:dbl)
          n504 = Divide(x=w1079, y=w1080) -> (x/y=→"DC Voltage":dbl)
          n505 = To Unsigned Word Integer(number=w1048) -> (unsigned 16bit integer=→"ECS State":u16)
          n506 = Subtract(x=w1043, y=50.0 ("x")) -> (x-y=→"Power transistor Heat sink Temp.":dbl)
          n507 = Subtract(x=w1045, y=50.0 ("x")) -> (x-y=→"Motor Stator Temp.":dbl)
          n508 = Equal?(x=u32 417408815, y=w1029) -> (x = y?=w1030:bool)
          n509 = Equal?(x=u32 417408831, y=w1029) -> (x = y?=w1032:bool)
          n510 = Equal?(x=u32 417408863, y=w1029) -> (x = y?=w1031:bool)
          n511 = Compound Arithmetic op=OR(w1032, w1031, w1030) -> (w1028:bool)
          n512 = case shown="True" w1028 {
            tunnel: w1041 -> [w1085 w1088]
            tunnel: [w1085 w1087] -> w1040
            tunnel: w1036 -> [_ w1086]
            frame False {
            }
            frame True {
              n513 = disable-structure shown="Disabled" {
                disable-tunnel: w1086 -> [w1092 _]
                frame Disabled {
                  n514 = call <vilib>:"Application Directory.vi"() -> ("Application Directory"=w1090:path)
                  n515 = Build Path(base path=w1090, name or relative path="RPM Log.lvm") -> (appended path=w1091:path)
                  n516 = call "Write To Measurement File"("Signals"=w1092, "Filename"=w1091) -> ()  [unwired: 15 in, 3 out]
                }
                frame Enabled {
                }
              }
              n517 = Build Array (concatenate)(w1086, w1088) -> (w1087:dbl[])
              "Waveform Chart" <- w1087
            }
          }
        }
        frame 1 {
          # "Framde ID\n0x18E3273F"
          n518 = control-ref of="UUT"() -> (w1093:refnum<vi>)
          n519 = property on="Property Node" class="DigNum (strict)"(reference=w1093) -> ("Value"=w1094:u8)  [unwired: 1 in, 2 out]
          n520 = Index Array(array=w1104, index #1=0 ("index"), index #2=1 ("index")) -> (element #1=w1102:u8, element #2=w1096:u8)
          n521 = Number To Boolean Array(number=w1102) -> (Boolean array=w1101:bool[])
          n522 = Number To Boolean Array(number=w1096) -> (Boolean array=w1098:bool[])
          n523 = Boolean To (0,1)(Boolean=w1098) -> (0, 1=w1095:i16[])
          n524 = Boolean To (0,1)(Boolean=w1101) -> (0, 1=w1100:i16[])
          n525 = case shown="95" w1094 {
            tunnel: w1095 -> [_ w1105]
            frame 0, Default {
            }
            frame 95 {
              n526 = for {
                tunnel: w1105 -> [w1110] mode=indexing
                i -> [w1106]
                stop <- w1108 stop-if-true
                n527 = Not Equal To 0?(x=w1110) -> (x != 0?=w1109:bool)
                n528 = case shown="0, Default" w1106 {
                  tunnel: w1109 -> [w1111 w1112]
                  frame 0, Default {
                    "Ambient Sensor temp" <- w1111
                  }
                  frame 1 {
                    "Ambient Over temp" <- w1112
                  }
                }
                n529 = Equal?(x=w1106, y=1.0) -> (x = y?=w1108:bool)
              }
            }
          }
          n530 = for {
            tunnel: w1100 -> [w1114] mode=indexing
            i -> [w1115]
            n531 = Not Equal To 0?(x=w1114) -> (x != 0?=w1113:bool)
            n532 = case shown="5" w1115 {
              tunnel: w1113 -> [w1116 w1117 w1118 w1119 w1120 w1121 w1122 w1123]
              frame 0, Default {
                "Drive Sensor temp Failure" <- w1116
              }
              frame 1 {
                "Drive Over temperature" <- w1117
              }
              frame 2 {
                "Motor Sensor temp Fauilre" <- w1118
              }
              frame 3 {
                "Motor Over temperature" <- w1119
              }
              frame 4 {
                "Derated drive temp" <- w1120
              }
              frame 5 {
                "Under voltage/Over voltage" <- w1121
              }
              frame 6 {
                "Commutation err" <- w1122
              }
              frame 7 {
                "Speed error" <- w1123
              }
            }
          }
        }
        frame 2 {
          # "Frame ID\n0x18E2273F"
          n533 = Index Array(array=w1136, index #1=0 ("index"), index #2=1 ("index")) -> (element #1=w1133:u8, element #2=w1129:u8)
          n534 = disable-structure shown="Enabled" {
            disable-tunnel: [w1139 w1140] -> w1134
            disable-tunnel: w1133 -> [w1138 w1140]
            frame Disabled {
              n535 = Number To Hexadecimal String(2:w1138) -> (0:w1137:string)  [unwired: 1 in]
              n536 = Hexadecimal String To Number(string=w1137) -> (number=w1139:u32)  [unwired: 2 in, 1 out]
            }
            frame Enabled {
            }
          }
          n537 = Number To Hexadecimal String(2:w1129) -> (0:w1127:string)  [unwired: 1 in]
          n538 = Hexadecimal String To Number(string=w1127) -> (number=w1128:u32)  [unwired: 2 in, 1 out]
          n539 = To Double Precision Float(number=w1128) -> (double precision float=w1125:dbl)
          n540 = To Double Precision Float(number=w1134) -> (double precision float=→"Motor Phase Current RMS":dbl)
          n541 = Subtract(x=w1125, y=50.0) -> (x-y=→"Ambient Temperature":dbl)
        }
      }
    }
  }
  n542 = while {
    shift-right: [w1158] -> _
    shift-left: T10."Initialize" -> [w1157]
    shift-right: [w1153] -> _
    shift-left: "" -> [w1152]
    shift-right: [w1154] -> _
    shift-left: w4 -> [w1155]
    shift-right: [w1151] -> _
    shift-left: _ -> [w1150]
    shift-right: [w1149] -> _
    shift-left: w8 -> [w1147]
    shift-right: [w1148] -> _
    shift-left: refnum<vi> refnum ("Config_CANAT") -> [w1146]
    shift-right: [w1144] -> _
    shift-left: w3 -> [w1145]
    stop <- w1156 stop-if-true
    n543 = case shown="\"MainProgram\"" w1157 {
      tunnel: [T10."MainProgram" T10."Stop" w1250 T10."Erase ATR Table"] -> w1158
      tunnel: [FALSE TRUE FALSE FALSE] -> w1156
      tunnel: [w1160 w1229 w1244 w1614] -> w1154
      tunnel: w1155 -> [_ w1210 w1248 _]
      tunnel: ["ATR Reset" "Program Stopped...\r\nPlease turn OFF All Power sinks" _ "Initialization State..."] -> w1153
      tunnel: [w1182 refnum<visa-resource-name> refnum ("VISA resource name") w1245 w1619] -> w1151
      tunnel: w1150 -> [w1182 w1226 w1246 _]
      tunnel: [w1169 refnum<queue> refnum ("queue out") w1240 w1612] -> w1149
      tunnel: [w1168 refnum<vi> refnum ("Config_CANAT") w1241 w1615] -> w1148
      tunnel: w1147 -> [w1169 w1230 w1243 w1612]
      tunnel: w1146 -> [w1168 _ w1242 _]
      tunnel: w1145 -> [w1167 w1220 w1239 w1611]
      tunnel: [w1167 refnum<queue> refnum ("queue out") w1238 w1611] -> w1144
      frame "Erase ATR Table", Default {
        w1163 = refnum<visa-resource-name> "COM4" ("VISA resource name")
        w1177 = FALSE ("Visible")
        n544 = property on="Serial Com" class="Bool"(error in=errorcluster {"status"=FALSE, "code"=0, "source"=""} ("error out"), "Visible"=TRUE) -> (error out=w1164:errorcluster)  [unwired: 1 in, 1 out]
        n545 = property on="VISA resource name" class="VISAName"(error in=w1164, "Visible"=w1177, "Value"=w1163) -> (error out=w1179:errorcluster)  [unwired: 1 in, 1 out]
        n546 = property on="VISA resource name" class="VISAName"(error in=w1164, "Value"=w1163) -> ()  [unwired: 1 in, 2 out]
        n547 = property on="Status" class="Bool (strict)"(error in=w1179, "Value"=w1177) -> (error out=w1172:errorcluster)  [unwired: 1 in, 1 out]
        n548 = flat-sequence {
          tunnel: [w1186] -> w1174
          tunnel: w1172 -> [w1184]
          tunnel: [w1184] -> w1171
          frame #0 {
            n549 = Two Button Dialog(message="Please seect the Unit Under Test.", 1:"AHU" ("F button name (\"Cancel\")"), 2:"EBAY" ("T button name (\"OK\")")) -> (T button?=w1186:bool)
          }
        }
        n550 = case shown="True" w1174 {
          tunnel: [string[][] [["6.1", "Visual Inspection", "", "", "", "", ""], ["6.1.1", "Verification of Components Not Installed", "N/A", "-", "", "", ""], ["", "", "", "", "", "", ""], ["6.1.2", "Manufacturing Defects", "N/A", "-", "", "", ""], ["", "", "", "", "", "", ""], ["6.2", "Power Supply Testing", "", "", "", "", ""], ["6.2.1", "Input Current Drawn", "", "", "", "", ""], ["6.2.1.1", "DC Input Current", "< 150", "-", "mA", "", ""], ["", "", "", "", "", "", ""], ["6.2.2", "Power Supply Voltages", "", "", "", "", ""], ["6.2.2.1", "12V", "12.0", "+/-0.500", "V", "", ""], ["6.2.2.2", "5V", "5.0", "+/-0.200", "V", "", ""], ["6.2.2.3", "3.3V", "3.3", "+/-0.100", "V", "", ""], ["6.2.2.4", "1.8V", "1.8", "+/-0.100", "V", "", ""], ["", "", "", "", "", "", ""], ["7", "Functional Test Procedure", "", "", "", "", ""], ["7.1", "Weight Check", "3800", "+/-100.0", "gr", "", ""], ["", "", "", "", "", "", ""], ["7.2", "Insulation Resistance Test", "", "", "", "", ""], ["7.2.1", "J3.B to Chassis", "> 1M", "-", "ohms", "", ""], ["7.2.2", "J1.16 to Chassis", "> 100K", "-", "ohms", "", ""], ["", "", "", "", "", "", ""], ["7.2", "Bonding Resistance", "", "", "", "", ""], ["7.2.3", "J1 Body to Chassis", "< 2m", "-", "ohms", "", ""], ["7.2.4", "J2  Body to Chassis", "< 2m", "-", "ohms", "", ""], ["7.2.5", "J3  Body to Chassis", "< 2m", "-", "ohms", "", ""], ["", "", "", "", "", "", ""], ["7.2.1", "CANbus Resistance Test", "", "", "", "", ""], ["7.2.1.1", "J1.17 to J1.18", "> 10K", "-", "ohms", "", ""], ["", "", "", "", "", "", ""], ["7.3", "Sealing Test", "N/A", "-", "", "", ""], ["", "", "", "", "", "", ""], ["7.4", "Communication Test", "", "", "", "", ""], ["7.4.1", "Serial RS-232", "N/A", "-", "", "", ""], ["7.4.2", "CAN Bus", "N/A", "-", "", "", ""], ["", "", "", "", "", "", ""], ["7.5", "Performances Tests", "", "", "", "", ""], ["7.5.1", "Reverse Polarity Test", "", "", "", "", ""], ["7.5.1.1", "DC Input Current", "< 1", "-", "mA", "", ""], ["", "", "", "", "", "", ""], ["7.5.2", "Enable Test", "", "", "", "", ""], ["7.5.2.1", "Fan Speed at Opened Enable ", "6000", "+/-200.0", "rpm", "", ""], ["7.5.2.2", "Fan Speed at Opened Enable ", "0", "+/-200.0", "rpm", "", ""], ["7.5.2.3", "Fan Speed at Closed Enable ", "6000", "+/-200.0", "rpm", "", ""], ["7.5.2.4", "Motor Rotation Direction", "Counter-clockwise (Inlet)", "-", "", "", ""], ["", "", "", "", "", "", ""], ["7.5.3", "Stop Time Test ", "", "", "", "", ""], ["7.5.3.1", "Motor Stop time", "< 50", "-", "sec", "", ""], ["", "", "", "", "", "", ""], ["7.5.4", "Speed Command Test", "", "", "", "", ""], ["7.5.4.1", "Fan Speed", "6000", "+/-200.0", "rpm", "", ""], ["7.5.4.2", "Fan Speed", "9000", "+/-200.0", "rpm", "", ""], ["7.5.4.3", "Fan Speed", "12100", "+/-200.0", "rpm", "", ""], ["", "", "", "", "", "", ""], ["7.5.5", "Temperature Sensor Calibration Test", "", "", "", "", ""], ["7.5.5.1", "Sensor Reading Analog Offset", "0", "+/-0.100", ".", "", ""], ["", "", "", "", "", "", ""], ["7.5.6", "Burn-in Test", "", "", "", "", ""], ["7.5.6.1", "DC Input Current", "28", "+/-5.000", "A", "", ""], ["7.5.6.2", "Ambient Temperature", "25", "+/-13.00", "Deg.", "", ""], ["7.5.6.3", "After 10 min of operation", "", "", "Deg.", "", ""], ["7.5.6.4", "After 20 min of operation", "", "", "Deg.", "", ""], ["7.5.6.5", "After 30 min of operation", "", "", "Deg.", "", ""], ["", "", "", "", "", "", ""], ["8", "Auxiliary", "", "", "", "", ""], ["8.1", "Auxiliary Cooling Fan 60 Deg", "On", "-", ".", "", ""], ["8.2", "Auxiliary Cooling Fan 55 Deg", "Off", "-", ".", "", ""]] ("data") string[][] [["6.1", "Visual Inspection", "", "", "", "", ""], ["6.1.1", "Verification of Components Not Installed", "N/A", "-", "", "", ""], ["", "", "", "", "", "", ""], ["6.1.2", "Manufacturing Defects", "N/A", "-", "", "", ""], ["", "", "", "", "", "", ""], ["6.2", "Power Supply Testing", "", "", "", "", ""], ["6.2.1", "Input Current Drawn", "", "", "", "", ""], ["6.2.1.1", "DC Input Current", "< 150", "-", "mA", "", ""], ["", "", "", "", "", "", ""], ["6.2.2", "Power Supply Voltages", "", "", "", "", ""], ["6.2.2.1", "12V", "12.0", "+/-0.500", "V", "", ""], ["6.2.2.2", "5V", "5.0", "+/-0.200", "V", "", ""], ["6.2.2.3", "3.3V", "3.3", "+/-0.100", "V", "", ""], ["6.2.2.4", "1.8V", "1.8", "+/-0.100", "V", "", ""], ["", "", "", "", "", "", ""], ["7", "Functional Test Procedure", "", "", "", "", ""], ["7.1", "Weight Check", "4180", "+/-10.00", "gr", "", ""], ["", "", "", "", "", "", ""], ["7.2", "Insulation Resistance Test", "", "", "", "", ""], ["7.2.1", "J3.B to Chassis", "> 1M", "-", "ohms", "", ""], ["7.2.2", "J1.16 to Chassis", "> 100K", "-", "ohms", "", ""], ["", "", "", "", "", "", ""], ["7.2", "Bonding Resistance", "", "", "", "", ""], ["7.2.3", "J1 Body to Chassis", "< 2m", "-", "ohms", "", ""], ["7.2.4", "J2  Body to Chassis", "< 2m", "-", "ohms", "", ""], ["7.2.5", "J3  Body to Chassis", "< 2m", "-", "ohms", "", ""], ["", "", "", "", "", "", ""], ["7.2.1", "CANbus Resistance Test", "", "", "", "", ""], ["7.2.1.1", "J1.17 to J1.18", "> 10K", "-", "ohms", "", ""], ["", "", "", "", "", "", ""], ["7.3", "Sealing Test", "N/A", "-", "", "", ""], ["", "", "", "", "", "", ""], ["7.4", "Communication Test", "", "", "", "", ""], ["7.4.1", "Serial RS-232", "N/A", "-", "", "", ""], ["7.4.2", "CAN Bus", "N/A", "-", "", "", ""], ["", "", "", "", "", "", ""], ["7.5", "Performances Tests", "", "", "", "", ""], ["7.5.1", "Reverse Polarity Test", "", "", "", "", ""], ["7.5.1.1", "DC Input Current", "< 1", "-", "mA", "", ""], ["", "", "", "", "", "", ""], ["7.5.2", "Enable Test", "", "", "", "", ""], ["7.5.2.1", "Fan Speed at Opened Enable ", "6000", "+/-200.0", "rpm", "", ""], ["7.5.2.2", "Fan Speed at Opened Enable ", "0", "+/-200.0", "rpm", "", ""], ["7.5.2.3", "Fan Speed at Closed Enable ", "6000", "+/-200.0", "rpm", "", ""], ["7.5.2.4", "Motor Rotation Direction", "Counter-clockwise (Inlet)", "-", "", "", ""], ["", "", "", "", "", "", ""], ["7.5.3", "Stop Time Test ", "", "", "", "", ""], ["7.5.3.1", "Motor Stop time", "< 50", "-", "sec", "", ""], ["", "", "", "", "", "", ""], ["7.5.4", "Speed Command Test", "", "", "", "", ""], ["7.5.4.1", "Fan Speed", "6000", "+/-200.0", "rpm", "", ""], ["7.5.4.2", "Fan Speed", "11500", "+/-200.0", "rpm", "", ""], ["7.5.4.3", "Fan Speed", "15100", "+/-200.0", "rpm", "", ""], ["", "", "", "", "", "", ""], ["7.5.5", "Temperature Sensor Calibration Test", "", "", "", "", ""], ["7.5.5.1", "Sensor Reading Analog Offset", "0", "+/-0.100", ".", "", ""], ["", "", "", "", "", "", ""], ["7.5.6", "Temperature Control Algorithm Test", "", "", "", "", ""], ["7.5.6.1", "Tair <   68 ± 2 oC", "6000", "+/-200.0", "rpm", "", ""], ["7.5.6.2", "Measured Temp.", "", "", "Deg.", "", ""], ["7.5.6.3", "Tair >= 68 ± 2 oC", "11500", "+/-200.0", "rpm", "", ""], ["7.5.6.4", "Transition Temp.", "", "", "Deg.", "", ""], ["7.5.6.5", "Tair >= 88 ± 2 oC", "15100", "+/-400.0", "rpm", "", ""], ["7.5.6.6", "Transition Temp.", "", "", "Deg.", "", ""], ["7.5.6.7", "Tair <= 80 ± 2 oC", "11500", "+/-200.0", "rpm", "", ""], ["7.5.6.8", "Transition Temp.", "", "", "Deg.", "", ""], ["7.5.6.9", "Tair <= 60 ± 2 oC", "6000", "+/-200.0", "rpm", "", ""], ["7.5.6.10", "Transition Temp.", "", "", "Deg.", "", ""], ["", "", "", "", "", "", ""], ["7.5.7", "Burn-in Test", "", "", "", "", ""], ["7.5.7.1", "DC Input Current", "50", "+/-5.000", "A", "", ""], ["7.5.7.2", "Fan Speed", "15100", "+/-400.0", "rpm", "", ""], ["7.5.7.3", "Ambient Temperature", "25", "+/-13.00", "Deg.", "", ""], ["7.5.7.4", "After 10 min of operation", "", "-", "Deg.", "", ""], ["7.5.7.5", "After 20 min of operation", "", "-", "Deg.", "", ""], ["7.5.7.6", "After 30 min of operation", "", "-", "Deg.", "", ""], ["", "", "", "", "", "", ""], ["8", "Auxiliary", "", "", "", "", ""], ["8.1", "Auxiliary Cooling Fan ON", "60", "+/-2.00", "Deg.", "", ""], ["8.2", "Fan status", "ON", "-", "-", "", ""], ["8.3", "Auxiliary Cooling Fan OFF", "55", "+/-2.00", "Deg.", "", ""], ["8.4", "Fan status", "OFF", "-", "-", "", ""]] ("data")] -> w1175
          tunnel: ["AHU" "EBAY"] -> w1173
          tunnel: [w1189 w1192] -> w1170
          tunnel: w1171 -> [w1189 w1192]
          frame False {
          }
          frame True {
          }
        }
        "UUT" <- w1173
        n551 = for {
          tunnel: w1175 -> [w1199] mode=indexing
          tunnel: w1170 -> [w1197]
          tunnel: [w1196] -> w1166
          tunnel: w1175 -> [w1195]
          i -> [w1198]
          n552 = for {
            tunnel: w1199 -> [_] mode=indexing
            tunnel: w1198 -> [w1205]
            tunnel: w1197 -> [w1202]
            tunnel: [w1201] -> w1196
            tunnel: w1195 -> [w1200]
            i -> [w1206]
            n553 = Bundle By Name(cluster=T12 {"Row"=0, "Column"=0} ("Active Cell:Active Cell"), "Row"=w1205, "Column"=w1206) -> (w1204:T12)
            n554 = control-ref of="ATR"() -> (w1203:refnum<vi>)
            n555 = property class="Tbl (strict)"(reference=w1203, error in=w1202, "Active Cell"=w1204, "Cell BG Color"=u32 16777226, "Value"=w1200) -> (error out=w1201:errorcluster)  [unwired: 1 out]
          }
        }
        n556 = call "COM EvolutionBoard.vi"("error in (no error)"=w1166, "VISA resource name 2"=refnum<visa-resource-name> "COM1" ("VISA resource name")) -> ("error out"=w1160:errorcluster, "VISA resource name out"=w1159:refnum<visa-resource-name>)  [unwired: 8 in]
        "VISA resource name out" <- w1159
        n557 = Byte Array To String(unsigned byte array=u8[] [75, 0, 4, 2, 0, 0, 2, 0] ("appended array")) -> (string=w1162:string)
        n558 = VISA Write(VISA resource name=w1159, write buffer=w1162, error in (no error)=w1160) -> ()  [unwired: 3 out]
      }
      frame "Stop" {
        # "K15 OFF + Venable"
        n559 = flat-sequence {
          tunnel: w1210 -> [w1235]
          tunnel: [w1234] -> w1209
          frame #0 {
            n560 = control-ref of="Pannel User Message"() -> (w1237:refnum<vi>)
            n561 = property class="Str"(reference=w1237, error in=w1235, "Value"="Program Stopped...\r\nPlease turn OFF All Power sinks") -> (error out=w1234:errorcluster)  [unwired: 1 out]
          }
        }
        n562 = control-ref of="VISA resource name out"() -> (w1218:refnum<vi>)
        n563 = property class="VISAName"(reference=w1218, error in=w1209) -> (error out=w1214:errorcluster, "Value"=w1213:refnum<visa-resource-name>)  [unwired: 1 out]
        n564 = Byte Array To String(unsigned byte array=u8[] [75, 0, 4, 2, 0, 0, 0, 0] ("appended array")) -> (string=w1216:string)
        n565 = VISA Close(VISA resource name=w1226, error in (no error)=w1209) -> (error out=w1219:errorcluster)
        n566 = VISA Write(VISA resource name=w1213, write buffer=w1216, error in (no error)=w1214) -> (VISA resource name out=w1212:refnum<visa-resource-name>, error out=w1211:errorcluster)  [unwired: 1 out]
        n567 = VISA Close(VISA resource name=w1212, error in (no error)=w1211) -> ()  [unwired: 1 out]
        n568 = Flush Queue(queue=w1220, error in (no error)=w1219) -> (queue out=w1222:refnum<queue>, error out=w1221:errorcluster)  [unwired: 1 out]
        n569 = Flush Queue(queue=w1230, error in (no error)=w1219) -> (queue out=w1227:refnum<queue>, error out=w1231:errorcluster)  [unwired: 1 out]
        n570 = Release Queue(queue=w1222, error in (no error)=w1221) -> ()  [unwired: 1 in, 3 out]
        n571 = Release Queue(queue=w1227, error in (no error)=w1231) -> (error out=w1229:errorcluster)  [unwired: 1 in, 2 out]
      }
      frame "MainProgram" {
        (unwired) "Main Program..."
        n572 = event shown="[0] Timeout" {
          selector: _ -> [_ _ _ _ _ _ _ _ _ _ _ _]
          dyn-events: _ -> [_ _ _ _ _ _ _ _ _ _ _ _]
          timeout: 50 -> [_ _ _ _ _ _ _ _ _ _ _ _]
          tunnel: [T10."MainProgram" T10."MainProgram" T10."MainProgram" T10."MainProgram" T10."Stop" T10."MainProgram" T10."MainProgram" T10."MainProgram" T10."MainProgram" T10."MainProgram" w1581 T10."MainProgram"] -> w1250
          tunnel: [w1251 w1318 w1324 w1332 w1346 w1349 w1505 w1519 w1531 w1536 w1586 w1595] -> w1244
          tunnel: w1248 -> [w1256 w1317 w1326 w1332 w1346 w1358 w1505 w1520 w1530 w1535 w1586 w1599]
          tunnel: [w1265 w1319 w1325 w1333 w1344 w1352 w1504 w1517 w1528 w1540 w1579 w1592] -> w1245
          tunnel: w1246 -> [w1265 w1319 w1325 w1333 w1344 w1352 w1504 w1517 w1528 _ w1579 w1592]
          tunnel: w1243 -> [w1258 w1313 w1321 w1329 w1343 w1355 w1469 w1516 w1527 w1544 w1578 w1591]
          tunnel: w1242 -> [w1252 w1314 w1322 w1330 w1342 w1356 w1468 w1515 w1526 w1543 w1577 w1590]
          tunnel: [w1254 w1314 w1322 w1330 w1342 w1356 w1468 w1515 w1526 w1543 w1577 w1590] -> w1241
          tunnel: [w1257 w1313 w1321 w1329 w1343 w1355 w1469 w1516 w1527 w1544 w1578 w1591] -> w1240
          tunnel: w1239 -> [w1255 w1312 w1320 w1328 w1341 w1354 w1467 w1514 w1525 w1542 w1576 w1589]
          tunnel: [w1255 w1312 w1320 w1328 w1341 w1348 w1467 w1514 w1525 w1542 w1576 w1589] -> w1238
          event Timeout {
            n573 = event-data() -> ()  [unwired: 1 in, 3 out]
            n574 = property class="Clust (strict)"(reference=w1252, error in=w1256) -> (reference out=w1254:refnum<vi>, error out=w1253:errorcluster, "Value"=w1262:T7)
            n575 = Unbundle By Name(w1262) -> ("DevType"=w1263:T2, "CanIndex"=w1260:T1)
            n576 = call "VCI_Receive.vi"("CANIndex"=w1260, "DevIndex"=u32 0, "DevType"=w1263) -> ("Recieve"=w1259:T17[])  [unwired: 3 in, 5 out]
            n577 = Empty Array?(array=w1259) -> (empty?=w1261:bool)
            n578 = case shown="False" w1261 {
              tunnel: w1260 -> [w1278 _]
              tunnel: w1254 -> [w1276 _]
              tunnel: w1258 -> [w1275 w1311]
              tunnel: w1253 -> [w1274 w1310]
              tunnel: w1259 -> [w1279 _]
              tunnel: [w1269 w1310] -> w1251
              tunnel: [w1268 w1311] -> w1257
              tunnel: [w1267 0] -> _
              frame False {
                n579 = call "Demo_MakeDispBuff.vi"("Channel"=w1278, "Type"=enum16{"接收", "发送"}."接收", "OBJs"=w1279) -> ("Buffer"=w1277:T18)
                n580 = for {
                  N: 3 -> [_]
                  tunnel: w1277 -> [w1293]
                  tunnel: w1276 -> [w1292]
                  tunnel: w1275 -> [w1283]
                  tunnel: w1274 -> [w1282]
                  tunnel: [w1285] -> w1272 mode=indexing
                  tunnel: [w1283] -> w1271
                  tunnel: [w1282] -> w1270
                  tunnel: [w1281] -> w1267
                  i -> [w1281]
                  n581 = property class="Clust (strict)"(reference=w1292) -> ("Value"=w1290:T7)  [unwired: 1 in, 2 out]
                  n582 = Index Array(array=w1293, index=w1281) -> (element=w1286:T19)
                  n583 = Unbundle By Name(w1286) -> ("Channel"=w1288:T1, "VCI_CAN_OBJ"=w1291:T17)  [unwired: 2 out]
                  n584 = Unbundle By Name(w1290) -> ("CanIndex"=w1289:T1)
                  n585 = Equal?(x=w1289, y=w1288) -> (x = y?=w1287:bool)
                  n586 = case shown="True" w1287 {
                    tunnel: w1291 -> [_ w1304]
                    tunnel: [w1294 w1300] -> w1285
                    tunnel: T13 {"ID"=0, "MSGTYPE"=0, "LEN"=0, "aDATA"=[]} ("Msg") -> [w1294 w1299]
                    frame False {
                    }
                    frame True {
                      n587 = Unbundle By Name(w1304) -> ("ID"=w1298:u32, "DataLen"=w1303:u8, "Data"=w1301:u8[])
                      n588 = Bundle By Name(cluster=w1299, "ID"=w1298, "MSGTYPE"=u8 0, "LEN"=w1303, "aDATA"=w1301) -> (w1300:T13)
                      n589 = Unbundle By Name(w1300) -> ("ID"=w1296:u32)
                      n590 = Split Number(x=w1296) -> (lo(x)=w1297:u16)  [unwired: 1 out]
                      n591 = Split Number(x=w1297) -> (lo(x)=w1295:u8)  [unwired: 1 out]
                      "UUT" <- w1295
                      n592 = case shown="63" w1295 {
                        tunnel: ["EBAY 5F" "" "AHU 3F" "AHU 2F"] -> _
                        frame 95 {
                        }
                        frame Default {
                        }
                        frame 63 {
                        }
                        frame 47 {
                        }
                      }
                    }
                  }
                }
                n593 = Enqueue Element(queue=w1271, element=w1272, error in (no error)=w1270) -> (queue out=w1268:refnum<queue>, error out=w1269:errorcluster)  [unwired: 2 out]
              }
              frame True {
              }
            }
          }
          event "ATR": Mouse Enter {
            n594 = event-data() -> ()  [unwired: 1 in, 4 out]
            n595 = call-poly <vilib>:"Set Cursor.vi"("error in (no error)"=w1317, "icon"=u16 1) -> ("error out"=w1318:errorcluster)  [unwired: 8 in, 1 out]
          }
          event "ATR": Mouse Leave {
            n596 = event-data() -> ()  [unwired: 1 in, 4 out]
            n597 = call-poly <vilib>:"Set Cursor.vi"("error in (no error)"=w1326, "icon"=u16 0) -> ("error out"=w1324:errorcluster)  [unwired: 8 in, 1 out]
          }
          event "ATR": Mouse Down? {
            n598 = event-data() -> ("Coords"=w1340:T20)  [unwired: 1 in, 4 out]
            n599 = invoke on="ATR" class="Tbl (strict)" method="Point To Row Column"("Point"=w1340) -> ("InBounds"=w1336:bool, "CellPosition"=w1335:T12)  [unwired: 5 in, 4 out]
            n600 = Greater Than 0?(x=w1335) -> (x > 0?=w1339:cluster{"Row":bool, "Column":bool})
            n601 = Cluster To Array(cluster=w1339) -> (array=w1338:bool[])
            n602 = Or Array Elements(Boolean array=w1338) -> (logical OR=w1337:bool)
            n603 = Or(x=w1336, y=w1337) -> (x .or. y?=w1334:bool)
            n604 = event-data("Discard?"=w1334) -> ()  [unwired: 1 in, 1 out]
          }
          event "Stop Button": Value Change {
            n605 = event-data() -> ()  [unwired: 1 in, 6 out]
          }
          event "Start": Value Change {
            n606 = event-data() -> ()  [unwired: 1 in, 2 out]
            n607 = property on="UUT" class="Str"(error in=w1358) -> ("Value"=w1357:string)  [unwired: 1 in, 2 out]
            n608 = case shown="\"AHU\", Default" w1357 {
              tunnel: [w1372 w1424] -> w1351
              tunnel: [w1371 w1423] -> w1350
              frame "AHU", Default {
                n609 = call "Load Program Process AHU.vi"() -> ("Speed Command Test"=w1364:bool, "Enable Test"=w1365:bool, "Burn-in Test"=w1362:bool, "Auxiliary"=w1360:bool, "Temperature Sensor Calibration Test"=w1367:bool, "Communication Test"=w1366:bool, "Stop Time Test"=w1363:bool, "Visual Inspection"=w1361:bool, "OK"=w1369:bool, "Automation"=w1368:bool, "error out"=w1371:errorcluster)  [unwired: 8 in, 9 out]
                n610 = Or(x=w1369, y=w1368) -> (x .or. y?=w1370:bool)
                n611 = case shown="True" w1370 {
                  tunnel: [w1373 w1383] -> w1372
                  tunnel: w1368 -> [_ w1382]
                  tunnel: w1367 -> [_ w1381]
                  tunnel: w1366 -> [_ w1380]
                  tunnel: w1365 -> [_ w1379]
                  tunnel: w1364 -> [_ w1378]
                  tunnel: w1363 -> [_ w1377]
                  tunnel: w1362 -> [_ w1376]
                  tunnel: w1361 -> [_ w1375]
                  tunnel: w1360 -> [_ w1374]
                  frame False {
                    w1373 = T21 [] items=["Visual Inspection", "Temp Sens Cal", "Com Test", "Enable Test", "Speed Command", "Stop Time", "Temp Control", "Burn in", "Visual Inspec", "Empty"]
                  }
                  frame True {
                    n612 = case shown="False" w1382 {
                      tunnel: [w1409 w1410] -> w1383
                      tunnel: w1381 -> [w1401 _]
                      tunnel: w1380 -> [w1400 _]
                      tunnel: w1379 -> [w1399 _]
                      tunnel: w1378 -> [w1398 _]
                      tunnel: w1377 -> [w1397 _]
                      tunnel: w1376 -> [w1396 _]
                      tunnel: w1375 -> [w1395 _]
                      tunnel: w1374 -> [w1387 _]
                      frame False {
                        w1386 = T14."Empty" ("f")
                        n613 = Select(t=T14."Temp Sens Cal" ("f"), s=w1401, f=w1386) -> (s? t:f=w1394:T14)
                        n614 = Select(t=T14."Com Test" ("f"), s=w1400, f=w1386) -> (s? t:f=w1393:T14)
                        n615 = Select(t=T14."Enable Test" ("f"), s=w1399, f=w1386) -> (s? t:f=w1392:T14)
                        n616 = Select(t=T14."Speed Command" ("f"), s=w1398, f=w1386) -> (s? t:f=w1391:T14)
                        n617 = Select(t=T14."Stop Time" ("f"), s=w1397, f=w1386) -> (s? t:f=w1390:T14)
                        n618 = Select(t=T14."Burn in" ("f"), s=w1396, f=w1386) -> (s? t:f=w1389:T14)
                        n619 = Select(t=T14."Auxiliary" ("f"), s=w1387, f=w1386) -> (s? t:f=w1384:T14)
                        n620 = Select(t=T14."Visual Inspec" ("f"), s=w1395, f=w1386) -> (s? t:f=w1388:T14)
                        n621 = Build Array(w1394, w1393, w1392, w1391, w1390, w1389, w1384, w1388) -> (w1409:T11)
                      }
                      frame True {
                        w1410 = T22 [enum."Temp Sens Cal", enum."Com Test", enum."Enable Test", enum."Speed Command", enum."Stop Time", enum."Burn in", enum."Auxiliary", enum."Visual Inspec"] items=["Auxiliary", "Temp Sens Cal", "Com Test", "Enable Test", "Speed Command", "Stop Time", "Burn in", "Visual Inspec", "Empty"]
                      }
                    }
                  }
                }
              }
              frame "EBAY" {
                n622 = call "Load Program Process EBAY.vi"() -> ("Speed Command Test"=w1416:bool, "Enable Test"=w1417:bool, "Burn-in Test"=w1414:bool, "Temperature Control Algorithm Test"=w1413:bool, "Auxiliary"=w1411:bool, "Temperature Sensor Calibration Test"=w1419:bool, "Communication Test"=w1418:bool, "Stop Time Test"=w1415:bool, "Visual Inspection"=w1412:bool, "OK"=w1421:bool, "Automation"=w1420:bool, "error out"=w1423:errorcluster)  [unwired: 8 in, 8 out]
                n623 = Or(x=w1421, y=w1420) -> (x .or. y?=w1422:bool)
                n624 = case shown="True" w1422 {
                  tunnel: [w1425 w1436] -> w1424
                  tunnel: w1420 -> [_ w1435]
                  tunnel: w1419 -> [_ w1434]
                  tunnel: w1418 -> [_ w1433]
                  tunnel: w1417 -> [_ w1432]
                  tunnel: w1416 -> [_ w1431]
                  tunnel: w1415 -> [_ w1430]
                  tunnel: w1414 -> [_ w1429]
                  tunnel: w1413 -> [_ w1428]
                  tunnel: w1412 -> [_ w1427]
                  tunnel: w1411 -> [_ w1426]
                  frame False {
                    w1425 = T11 [] items=["Auxiliary", "Temp Sens Cal", "Com Test", "Enable Test", "Speed Command", "Stop Time", "Temp Control", "Burn in", "Visual Inspec", "Empty"]
                  }
                  frame True {
                    n625 = case shown="False" w1435 {
                      tunnel: [w1465 w1466] -> w1436
                      tunnel: w1434 -> [w1456 _]
                      tunnel: w1433 -> [w1455 _]
                      tunnel: w1432 -> [w1454 _]
                      tunnel: w1431 -> [w1453 _]
                      tunnel: w1430 -> [w1452 _]
                      tunnel: w1429 -> [w1438 _]
                      tunnel: w1428 -> [w1437 _]
                      tunnel: w1427 -> [w1451 _]
                      tunnel: w1426 -> [w1442 _]
                      frame False {
                        w1440 = T14."Empty" ("f")
                        n626 = Select(t=T14."Temp Sens Cal" ("f"), s=w1456, f=w1440) -> (s? t:f=w1450:T14)
                        n627 = Select(t=T14."Com Test" ("f"), s=w1455, f=w1440) -> (s? t:f=w1449:T14)
                        n628 = Select(t=T14."Enable Test" ("f"), s=w1454, f=w1440) -> (s? t:f=w1448:T14)
                        n629 = Select(t=T14."Speed Command" ("f"), s=w1453, f=w1440) -> (s? t:f=w1447:T14)
                        n630 = Select(t=T14."Stop Time" ("f"), s=w1452, f=w1440) -> (s? t:f=w1446:T14)
                        n631 = Select(t=T14."Temp Control" ("f"), s=w1437, f=w1440) -> (s? t:f=w1445:T14)
                        n632 = Select(t=T14."Burn in" ("f"), s=w1438, f=w1440) -> (s? t:f=w1444:T14)
                        n633 = Select(t=T14."Visual Inspec" ("f"), s=w1451, f=w1440) -> (s? t:f=w1443:T14)
                        n634 = Select(t=T14."Auxiliary" ("f"), s=w1442, f=w1440) -> (s? t:f=w1439:T14)
                        n635 = Build Array(w1450, w1449, w1448, w1447, w1446, w1445, w1444, w1439, w1443) -> (w1465:T11)
                      }
                      frame True {
                        w1466 = T11 [enum."Temp Sens Cal", enum."Com Test", enum."Enable Test", enum."Speed Command", enum."Stop Time", enum."Temp Control", enum."Burn in", enum."Auxiliary", enum."Visual Inspec"] items=["Auxiliary", "Temp Sens Cal", "Com Test", "Enable Test", "Speed Command", "Stop Time", "Temp Control", "Burn in", "Visual Inspec", "Empty"]
                      }
                    }
                  }
                }
              }
            }
            n636 = Bundle By Name(cluster=T8 {"VISA"="COM1", "Array Test"=[]}, "VISA"=w1352, "Array Test"=w1351) -> (w1347:T8)
            n637 = Enqueue Element(queue=w1354, element=w1347, error in (no error)=w1350) -> (queue out=w1348:refnum<queue>, error out=w1349:errorcluster)  [unwired: 2 out]
          }
          event "Report": Value Change {
            n638 = event-data() -> ()  [unwired: 1 in, 6 out]
            n639 = call <vilib>:"Application Directory.vi"() -> ("Application Directory"=w1483:path)
            n640 = Build Path(base path=w1483, name or relative path="Reports") -> (appended path=w1486:path)
            n641 = local read "UUT"() -> (w1470:string)
            n642 = call <vilib>:"Check if File or Folder Exists.vi"("path"=w1486) -> ("error out"=w1484:errorcluster, "file or folder exists?"=w1487:bool, "dup path"=w1485:path)  [unwired: 8 in]
            n643 = control-ref of="ATR"() -> (w1501:refnum<vi>)
            n644 = case shown="False" w1487 {
              tunnel: w1484 -> [w1511 w1512]
              tunnel: w1485 -> [w1510 w1513]
              tunnel: [w1509 w1513] -> w1499
              tunnel: [w1508 w1512] -> w1493
              frame False {
                n645 = Create Folder(path (use dialog)=w1510, error in=w1511) -> (created path=w1509:path, error out=w1508:errorcluster)  [unwired: 1 in, 1 out]
              }
              frame True {
              }
            }
            n646 = Get Date/Time String(want seconds? (F)=TRUE) -> (date string=w1491:string, time string=w1490:string)  [unwired: 2 in]
            n647 = property on="Logger Path" class="Path"(error in=w1493, "Value"=w1499, "StartPath"=w1499) -> (error out=w1494:errorcluster)  [unwired: 1 in, 1 out]
            n648 = Search and Replace String(replace all?=TRUE ("replace all? (F)"), input string=w1491, search string="/") -> (result string=w1489:string)  [unwired: 5 in, 3 out]
            n649 = Search and Replace String(replace all?=TRUE ("replace all? (F)"), input string=w1490, search string=":") -> (result string=w1488:string)  [unwired: 5 in, 3 out]
            n650 = call "HeaderuRayon.vi"("UUT"=w1470) -> ("HEADER1"=w1500:string)  [unwired: 2 in]
            n651 = call <vilib>:"Space Constant.vi"() -> ("String"=w1471:string)
            n652 = Concatenate Strings(w1489, w1471, w1488, w1471, w1470, w1471, "Report.docx" ("string")) -> (w1473:string)
            n653 = property on="Logger Path" class="Path"(error in=w1494) -> (error out=w1495:errorcluster, "StartPath"=w1492:path)  [unwired: 1 in, 1 out]
            n654 = Build Path(base path=w1492, name or relative path=w1473) -> (appended path=w1474:path)
            n655 = call <vilib>:"Check if File or Folder Exists.vi"("error in (no error)"=w1495, "path"=w1474) -> ("error out"=w1496:errorcluster, "file or folder exists?"=w1497:bool)  [unwired: 7 in, 1 out]
            n656 = case shown="True" w1497 {
              tunnel: [T15."create" ("operation (0:open)") T15."replace" ("operation (0:open)")] -> w1498
              frame False {
              }
              frame True {
              }
            }
            n657 = Open/Create/Replace File(file path (use dialog)=w1474, error in=w1496, operation (0:open)=w1498) -> (error out=w1475:errorcluster)  [unwired: 3 in, 2 out]
            n658 = property class="Tbl (strict)"(reference=w1501, error in=w1475) -> ("Value"=w1502:string[][])  [unwired: 2 out]
            n659 = call "MarvinReport.vi"("HEADER1"=w1500, "ATR Or"=w1501, "Steps   pfull"=w1502, "pageNum"=3, "FILE NAME"=w1473, "Report Folder"=w1474) -> ()  [unwired: 8 in, 2 out]
          }
          event "Help Button": Value Change {
            n660 = event-data() -> ()  [unwired: 1 in, 6 out]
            n661 = vi-ref "Help.vi"() -> (w1522:refnum<vi>)
            n662 = invoke class="VI" method="FP.Open"(reference=w1522, error in=w1520, "Activate"=TRUE ("Activate?"), "State"=T16."Standard") -> (error out=w1521:errorcluster)  [unwired: 1 in, 4 out]
            n663 = call "Help.vi"("error in"=w1521) -> ("error out"=w1519:errorcluster)  [unwired: 7 in]
          }
          event "Serial Com": Value Change {
            n664 = event-data() -> ()  [unwired: 1 in, 6 out]
            n665 = property on="Serial Com" class="Bool"(error in=w1530, "Visible"=FALSE) -> (error out=w1534:errorcluster)  [unwired: 1 in, 1 out]
            n666 = property on="VISA resource name" class="VISAName"(error in=w1534, "Visible"=TRUE) -> (error out=w1531:errorcluster)  [unwired: 1 in, 1 out]
          }
          event "VISA resource name": Value Change {
            n667 = event-data() -> ()  [unwired: 1 in, 6 out]
            n668 = control-ref of="This VI"() -> (w1549:refnum<vi>)
            n669 = property on="Pannel User Message" class="Str"(error in=w1535, "Value"="Serial conection in process" ("Pannel User Message")) -> ()  [unwired: 1 in, 2 out]
            n670 = call "Serial InitMarvin.vi"("error in (no error)"=w1535, "VI reference (current VI)"=w1549, "VISA Refnum in"="VISA resource name") -> ("error out"=w1556:errorcluster, "Boolean"=w1541:bool)  [unwired: 7 in]
            n671 = property on="Status" class="Bool (strict)"(error in=w1556, "Value"=w1541) -> (error out=w1553:errorcluster)  [unwired: 1 in, 1 out]
            n672 = property on="VISA resource name" class="VISAName"(error in=w1553, "Visible"=FALSE) -> (error out=w1552:errorcluster)  [unwired: 1 in, 1 out]
            n673 = property on="Serial Com" class="Bool"(error in=w1552, "Visible"=TRUE) -> (error out=w1548:errorcluster)  [unwired: 1 in, 1 out]
            n674 = call "Serial.vi"("error in (no error)"=w1548, "Clear Log"=FALSE, "VISA resource name"="VISA resource name") -> ("error out"=w1547:errorcluster)  [unwired: 7 in, 1 out]
            n675 = call <vilib>:"Clear Errors.vi"("error in (no error)"=w1547) -> ("error out"=w1557:errorcluster)  [unwired: 5 in, 1 out]
            n676 = case shown="True" w1541 {
              tunnel: w1557 -> [w1571 w1575]
              tunnel: [w1571 w1574] -> w1539
              tunnel: "VISA resource name" -> [w1570 w1573]
              tunnel: [w1570 w1572] -> w1540
              frame False {
              }
              frame True {
                n677 = VISA Flush I/O Buffer(VISA resource name=w1573, error in (no error)=w1575) -> (VISA resource name out=w1572:refnum<visa-resource-name>, error out=w1574:errorcluster)  [unwired: 1 in]
              }
            }
            n678 = call "Display Message to User2"("error in (no error)"=w1539) -> ("error out"=w1538:errorcluster, "Yes"=w1537:bool)  [unwired: 9 in]
            n679 = case shown="True" w1537 {
              tunnel: w1538 -> [w1558 w1562]
              tunnel: [w1558 w1561] -> w1536
              frame False {
              }
              frame True {
                n680 = property on="Status" class="Bool (strict)"() -> ("Value"=w1560:bool)  [unwired: 2 in, 2 out]
                n681 = property on="VISA resource name" class="VISAName"() -> ("Value"=w1559:refnum<visa-resource-name>)  [unwired: 2 in, 2 out]
                n682 = case shown="True" w1560 {
                  selector: w1560 -> [_ w1566]
                  tunnel: w1562 -> [w1564 w1569]
                  tunnel: w1559 -> [_ w1568]
                  tunnel: [w1563 w1567] -> w1561
                  frame False {
                    n683 = call "Display Message to User3"("error in (no error)"=w1564) -> ("error out"=w1563:errorcluster)  [unwired: 9 in, 1 out]
                  }
                  frame True {
                    n684 = property on="UUT" class="DigNum (strict)"() -> ("Value"=w1565:u8)  [unwired: 2 in, 2 out]
                    n685 = call "SetParam.vi"("RS"=w1566, "error in (no error)"=w1569, "Param to Set in"=w1565, "Visa"=w1568) -> ("error out"=w1567:errorcluster)  [unwired: 7 in]
                  }
                }
              }
            }
          }
          event "Refresh Button": Value Change {
            n686 = event-data() -> ()  [unwired: 1 in, 6 out]
            n687 = property on="Refresh Button" class="Bool (strict)"("Value"=FALSE ("Refresh Button")) -> ()  [unwired: 2 in, 2 out]
            n688 = Two Button Dialog(message="Do you want to erase ATR table?", 1:"No" ("F button name (\"Cancel\")"), 2:"Yes" ("T button name (\"OK\")")) -> (T button?=w1582:bool)
            n689 = case shown="False" w1582 {
              tunnel: [T10."Initialize" T10."Erase ATR Table"] -> w1581
              frame False {
              }
              frame True {
              }
            }
          }
          event "Settings": Value Change {
            n690 = event-data() -> ()  [unwired: 1 in, 6 out]
            n691 = call "Settings"("error in (no error)"=w1599) -> ("Password"=w1598:string, "error out"=w1596:errorcluster)  [unwired: 16 in, 1 out]
            n692 = Equal?(x=w1598, y="123") -> (x = y?=w1594:bool)
            n693 = case shown="True" w1594 {
              tunnel: w1596 -> [w1600 w1607]
              tunnel: [w1600 w1605] -> w1595
              frame False {
                n694 = One Button Dialog(message="Wrong Password!") -> ()  [unwired: 1 in, 1 out]
              }
              frame True {
                n695 = vi-ref "Write Configuration (INI) File.vi"() -> (w1604:refnum<vi>)
                n696 = invoke class="VI" method="FP.Open"(reference=w1604, error in=w1607, "Activate"=TRUE ("Activate?"), "State"=T16."Standard") -> (error out=w1606:errorcluster)  [unwired: 1 in, 4 out]
                n697 = call "Write Configuration (INI) File.vi"("error in"=w1606) -> ("error out"=w1605:errorcluster)  [unwired: 10 in]
              }
            }
          }
        }
      }
      frame "Initialize" {
        w1619 = refnum<visa-resource-name> "COM1" ("VISA resource name")
        w1608 = FALSE ("Visible")
        n698 = disable-structure shown="Disabled" {
          frame Disabled {
            n699 = local write "UUT"("" ("UUT")) -> ()
          }
          frame Enabled {
          }
        }
        n700 = property on="Serial Com" class="Bool"(error in=errorcluster {"status"=FALSE, "code"=0, "source"=""} ("error out"), "Visible"=TRUE) -> (error out=w1623:errorcluster)  [unwired: 1 in, 1 out]
        n701 = property on="VISA resource name" class="VISAName"(error in=w1623, "Visible"=w1608, "Value"=w1619) -> (error out=w1610:errorcluster)  [unwired: 1 in, 1 out]
        n702 = property on="Stop Burn-in" class="Bool"(error in=w1610, "Visible"=w1608) -> (error out=w1609:errorcluster)  [unwired: 1 in, 1 out]
        n703 = flat-sequence {
          tunnel: w1609 -> [w1627]
          tunnel: [w1626] -> w1617
          tunnel: [w1629] -> w1616
          tunnel: w1617 -> [w1629]
          tunnel: [w1642] -> w1615
          tunnel: w1616 -> [w1643]
          tunnel: [w1643] -> w1614
          frame #0 {
            n704 = control-ref of="This VI"() -> (w1628:refnum<vi>)
            n705 = invoke class="VI" method="Default Vals.Reinit All"(reference=w1628, error in=w1627) -> (error out=w1626:errorcluster)  [unwired: 1 in, 2 out]
          }
          frame #1 {
            w1633 = u32 4294967295  # AccMask
            w1632 = T4 0 items=["使用Flash参数", "使用界面设置参数"] ("InitFlag")
            w1630 = T6 0 items=["normal operation", "Listen-only mode", "test mode"]  # Mode
            w1631 = T5 3 items=["接收所有类型"=1, "只接收标准帧"=2, "只接收扩展帧"=3] ("Fliter")
            w1637 = u8 10 items=["5k bps"=1, "10k bps"=2, "20k bps"=3, "40k bps"=4, "50k bps"=5, "80k bps"=6, "100k bps"=7, "125k bps"=8, "200k bps"=9, "250k bps"=10, "400k bps"=11, "500k bps"=12, "666k bps"=13, "800k bps"=14, "1000k bps"=15, "33.33k bps"=16, "66.66k bps"=17, "83.33k bps"=18]  # kBaudRate
            w1634 = u32 0  # AccCode
            w1635 = T2 4 items=["USB-CAN"=3, "USB-CAN2"=4] ("DevType")
            w1636 = T7 {"DevType"=3, "DevIndex"=0, "CanIndex"=0, "VCI_INIT_CONFIG"={"AccCode"=0, "AccMask"=0, "InitFlag"=1, "Fliter"=7, "Timing0"=0, "Timing1"=0, "Mode"=0}}  # Config
            # "CANalystII"
            n706 = call "Demo_GetT0T1.vi"("kBaudRate"=w1637) -> ("Timing0"=w1639:u8, "Timing1"=w1640:u8)
            n707 = Bundle By Name(cluster=w1636, "DevType"=w1635, "CanIndex"="Channel 2", "VCI_INIT_CONFIG.AccCode"=w1634, "VCI_INIT_CONFIG.AccMask"=w1633, "VCI_INIT_CONFIG.InitFlag"=w1632, "VCI_INIT_CONFIG.Fliter"=w1631, "VCI_INIT_CONFIG.Timing0"=w1639, "VCI_INIT_CONFIG.Timing1"=w1640, "VCI_INIT_CONFIG.Mode"=w1630) -> (→"Config_CANAT":T7)
          }
          frame #2 {
            w1644 = u16 284 items=["1M"=20, "500K"=28, "250K"=284, "125K"=796, "100K"=17199, "50K"=18223, "20K"=21295, "10K"=26415, "5K"=32639] ("baud in")
            n708 = control-ref of="Config_CANAT"() -> (w1642:refnum<vi>)
            n709 = call "InitCAN_ATII.vi"("Config"=w1642) -> ("Sts"=→"CAN Status":bool)
            n710 = call "ChangeCANBaud.vi"("baud in"=w1644, "reference"=w1642) -> ()
          }
        }
        n711 = Wait (ms)(milliseconds to wait=u32 500) -> ()  [unwired: 1 out]
        "Status" <- FALSE ("Serial Status")
      }
    }
    "Pannel User Message" <- w1152
  }
  n712 = disable-structure shown="Disabled" {
    frame Disabled {
      (unwired) 5 ("disabled index (col)")
      (unwired) 3 ("index (row)")
      (unwired) 4 ("disabled index (col)")
      (unwired) 3 ("index (row)")
      n713 = property class="Tbl (strict)"() -> (reference out=w1649:refnum<vi>, error out=w1650:errorcluster, "Value"=w1652:string[][])  [unwired: 2 in]
      n714 = Replace Array Subset(array=w1652) -> (w1651:string[][])  [unwired: 3 in]
      n715 = property class="Tbl (strict)"(reference=w1649, error in=w1650, "Value"=w1651) -> (reference out=w1647:refnum<vi>, error out=w1648:errorcluster)
      n716 = call "PassOrFail (SubVI).vi"("error in (no error)"=w1648, "Table in"=w1647) -> ()  [unwired: 9 in, 1 out]
    }
    frame Enabled {
    }
  }
  n717 = disable-structure shown="Disabled" {
    frame Disabled {
      (unwired) 0.5 ("Delay Time (sec)")
      n718 = call <vilib>:"Set Busy.vi"() -> ()  [unwired: 10 in, 2 out]
      n719 = call <vilib>:"Unset Busy.vi"() -> ()  [unwired: 11 in, 1 out]
      n720 = call <vilib>:"Clear Errors.vi"() -> ()  [unwired: 6 in, 2 out]
      n721 = call "Wait_Sec.vi"() -> ()  [unwired: 4 in, 1 out]
    }
    frame Enabled {
    }
  }
  n722 = disable-structure shown="Disabled" {
    frame Disabled {
      n723 = case shown="\" float\"" {
        selector: _ -> [_ _]
        tunnel: [u32 0 ("Data I") w1655] -> _
        frame "Int", Default {
        }
        frame " float" {
          n724 = To Single Precision Float(number=sgl 0.0 ("Data F")) -> (single precision float=w1657:sgl)
          n725 = call "Int_Float.vi"("1 Float in"=w1657) -> ("1 Int out"=w1656:i32)  [unwired: 1 in, 1 out]
          n726 = To Unsigned Long Integer(number=w1656) -> (unsigned 32bit integer=w1655:u32)
        }
      }
    }
    frame Enabled {
    }
  }
  n727 = disable-structure shown="Disabled" {
    frame Disabled {
      n728 = control-ref of="ATR"() -> (w1659:refnum<vi>)
      n729 = call "Table_Put_Resultes_and_Decided_Pass_Fail.vi"("Table Ref."=w1659) -> ("Table Out"=→"Table Out":string[][])  [unwired: 11 in, 3 out]
    }
    frame Enabled {
    }
  }
